vi "曲线.vi"() -> ()   [LabVIEW 2020]
uses:
  Global_Variable/Global.vi
  Database/Global1.vi
  Global_Variable/A131258.vi
  <vilib>/addons/database/Connection.llb/DB Tools Open Connec (String).vi
  <vilib>/addons/database/Connection.llb/Conn Execute.vi
  <vilib>/addons/database/Recordset.llb/Rec Fetch Recordset Data (R).vi
  <vilib>/Utility/config.llb/NI_LVConfig.lvlib
  <vilib>/addons/database/NI_Database_API.lvlib
panel:
  out "CODE_ID":string
  out "联机模式":string
  out "用户权限":string
  out "用户名":string
  in  "报表":string[][](table)=[["mm"], ["mm/s"]]
  in  "判定结果 3":bool[][](array[boolean])=[[TRUE]]
  in  "选项卡控件 2":enum32{"左工位压装曲线", "右工位压装曲线 ", "参数查看"}(tab)
  out "左压装下限":dbl format="%#.2f"
  out "左压装上限":dbl format="%#.2f"
  out "左下限2":dbl format="%#.2f"
  out "左上限2":dbl format="%#.2f"
  out "左下限1":dbl format="%#.2f"
  out "左上限1":dbl format="%#.2f"
  out "压装最大位移(mm)":dbl
  out "判定结果":bool
  out "力位移曲线":cluster{dbl[], dbl[]}[](graph)
  out "位移区间最大压力(KN)":dbl
  out "位移区间最小压力(KN)":dbl
  out "右位移下限":dbl format="%#.2f"
  out "右位移上限":dbl format="%#.2f"
  out "右下限2":dbl format="%#.2f"
  out "右上限2":dbl format="%#.2f"
  out "右下限1":dbl format="%#.2f"
  out "右上限1":dbl format="%#.2f"
  out "压装最大位移(mm) 2":dbl
  out "判定结果 2":bool
  out "力位移曲线 2":cluster{dbl[], dbl[]}[](graph)
  out "位移区间最大压力(KN) 2":dbl
  out "位移区间最小压力(KN) 2":dbl
  in  "删除":bool
  in  "确定":bool
  in  "添加":bool
  in  "退出":bool
  in  "更新":bool
  in  "产品型号":string(combo)
  in  "选项卡控件 3":enum32{"左工位参数", "右工位参数", "产品管理", "用户管理"}(tab)
  in  "左工位坐标轴参数":string[][](table)=[["mm"], ["mm/s"]]
  in  "左工位判定框参数":string[][](table)=[["mm"], ["mm/s"]]
  in  "左工位结果判定参数":string[][](table)=[["mm"], ["mm/s"]]
  in  "右工位结果判定参数":string[][](table)=[["mm"], ["mm/s"]]
  in  "右工位判定框参数":string[][](table)=[["mm"], ["mm/s"]]
  in  "右工位坐标轴参数":string[][](table)=[["mm"], ["mm/s"]]
  in  "请输入添加的产品名称":string
  in  "请选择要删除的产品":string(combo)
  in  "确定按钮":bool
  # "180上下柱管总成装配"
  # "上限"
  # "下限"
  # "上限"
  # "下限"
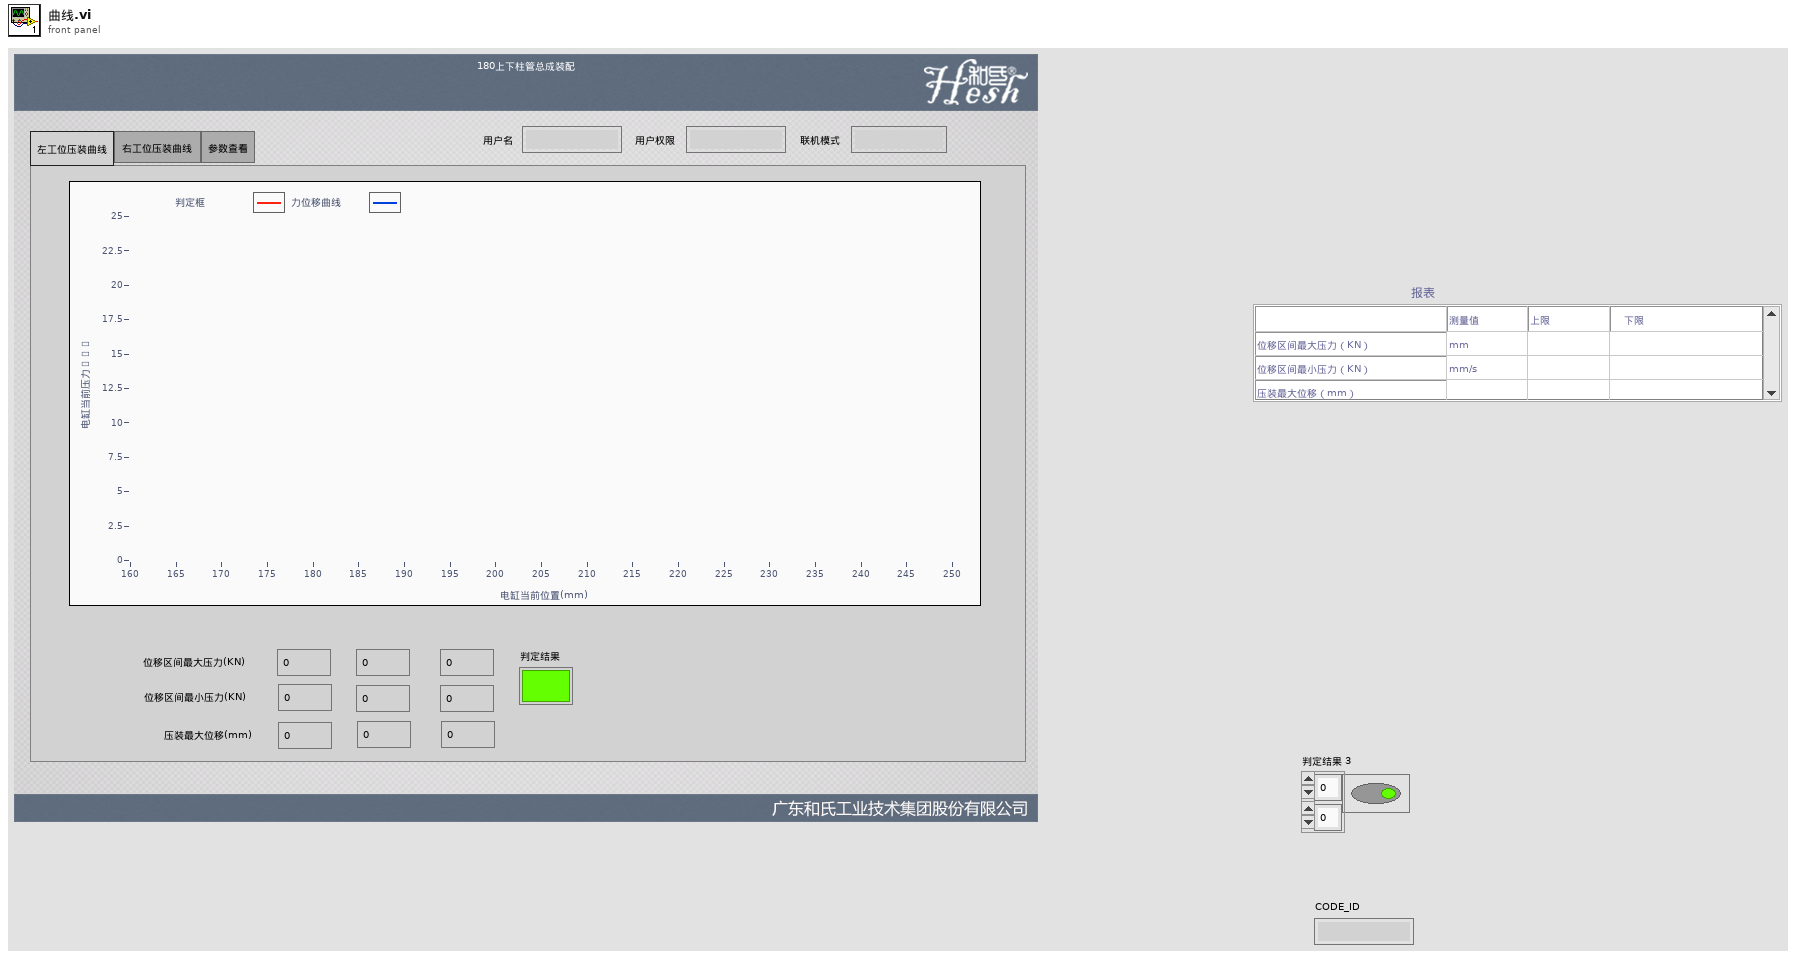
[diagram p1: front panel]
types:
  T1 = enum32{"Invalid", "Standard", "Closed", "Hidden", "Minimized", "Maximized"}
  T2 = cluster{"用户编号":string, "用户名":string, "用户密码(密文)":string, "用户权限":string}
  T3 = cluster{"设备名称":string, "用户名":string, "设备状态":enum16{"设备离线", "设备正常", "设备缺料", "设备故障", "质量报警"}, "附加信息":string}
  T4 = typedef "NI_LVConfig.lvlib/Config Data RefNum.ctl" = refnum<k1>
  T5 = typedef "NI_Database_API.lvlib/Conn ObjectReference.ctl" = refnum<k1>
  T6 = typedef "NI_Database_API.lvlib/Rec ObjectReference.ctl" = refnum<k1>
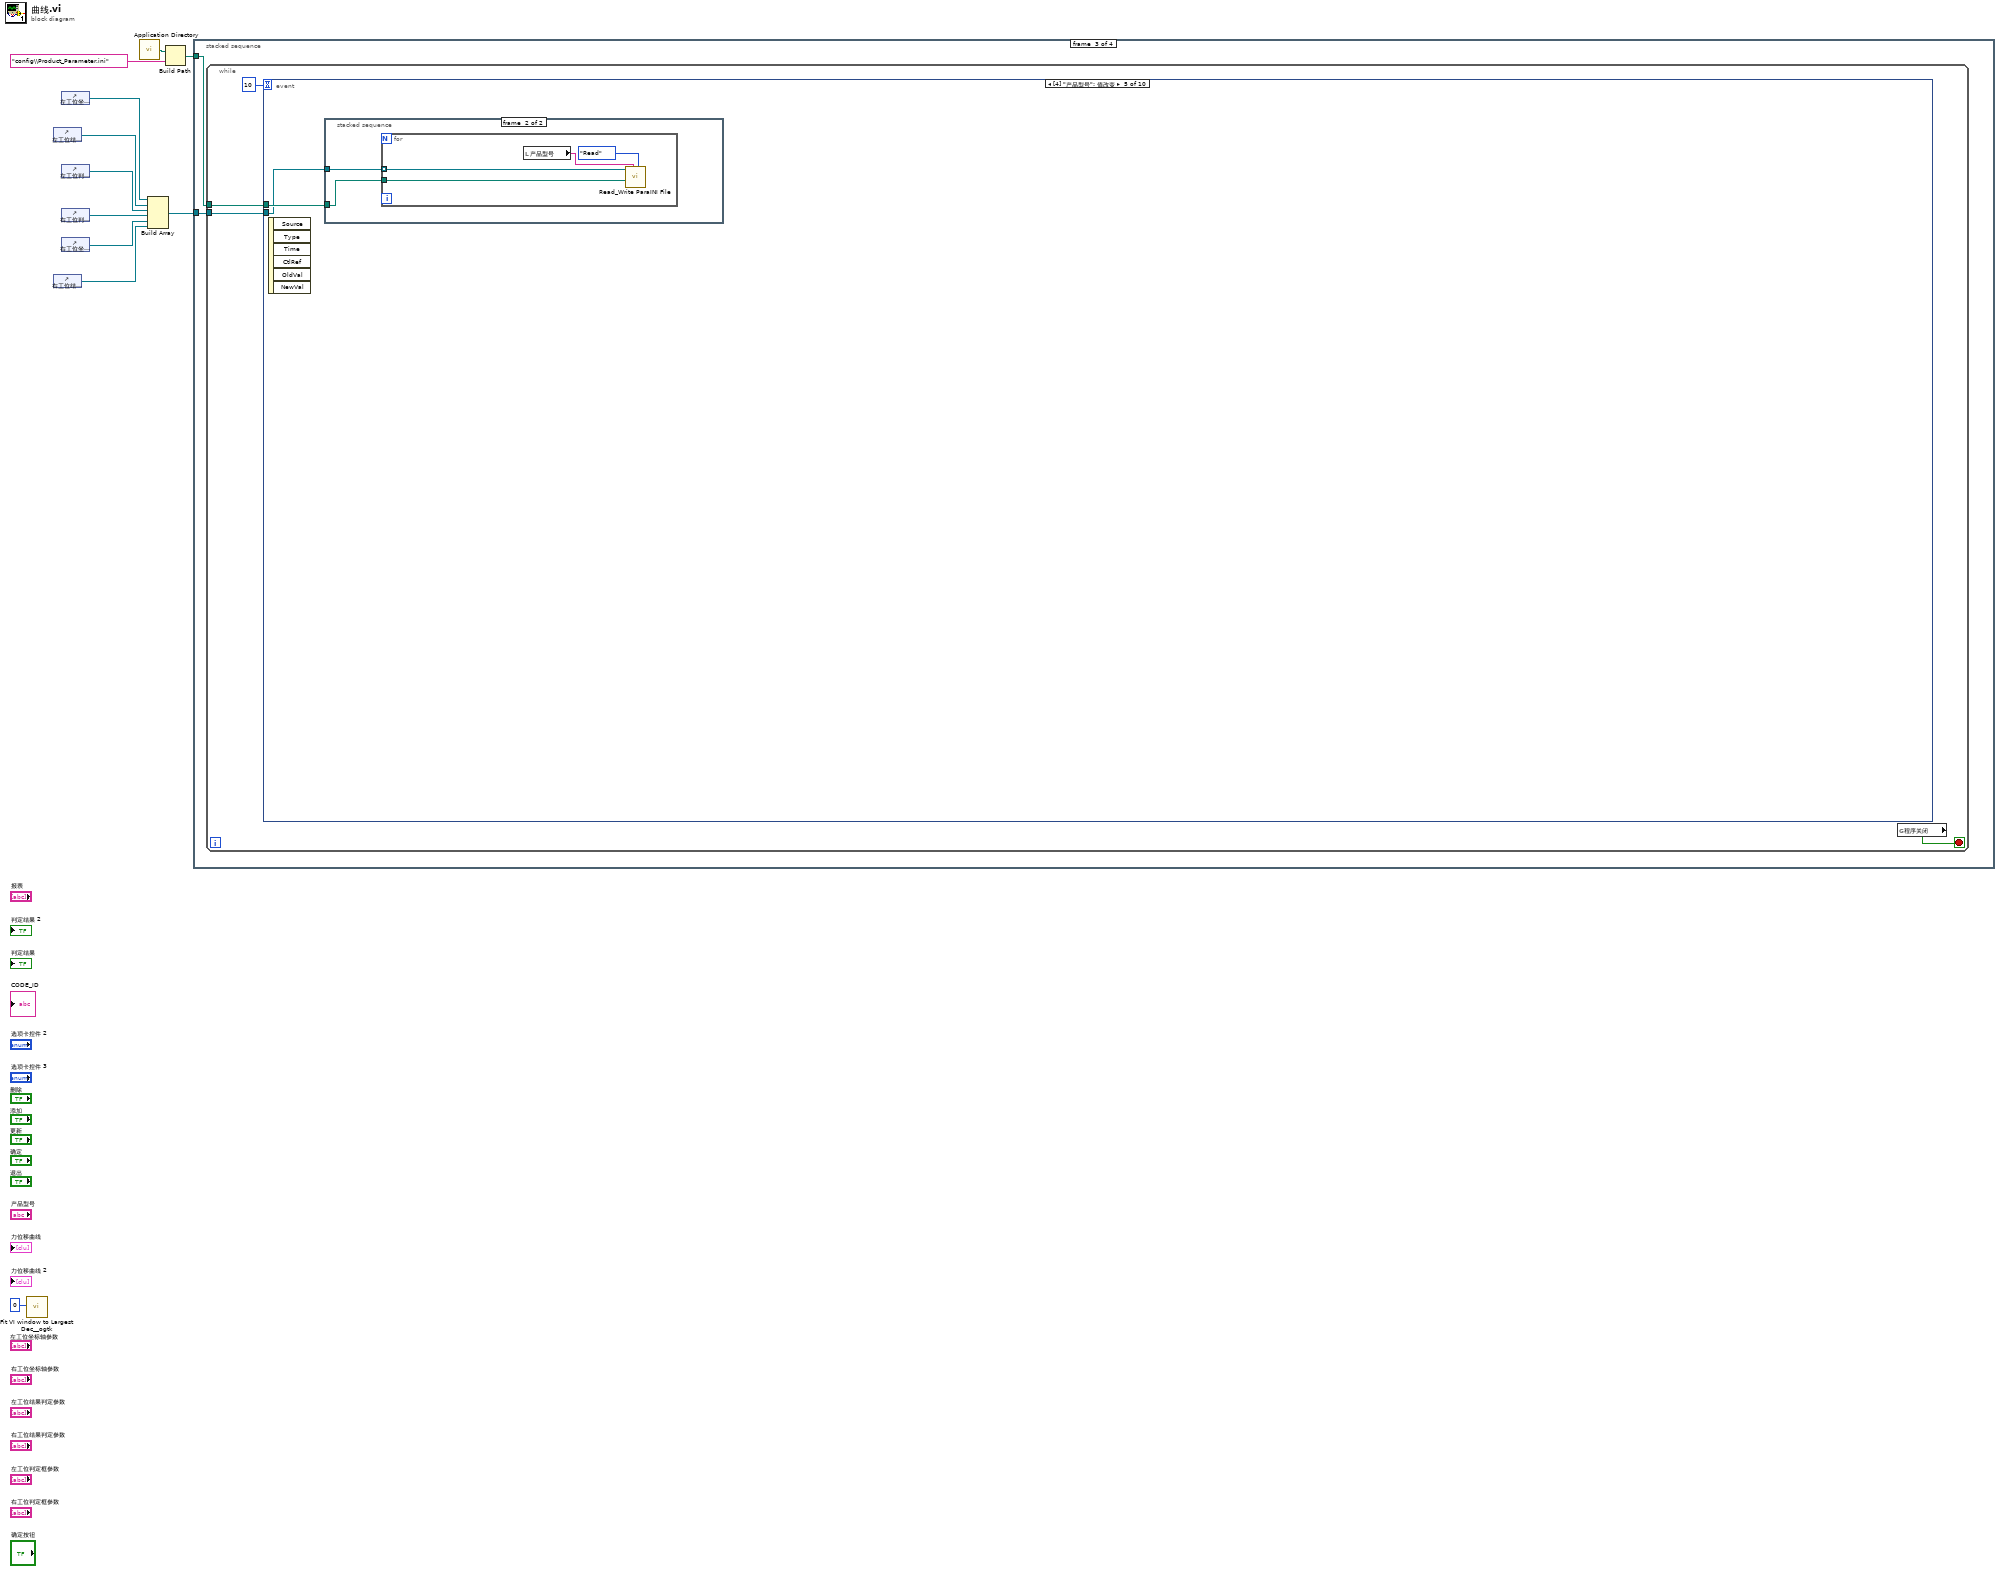
[diagram p0: block diagram]
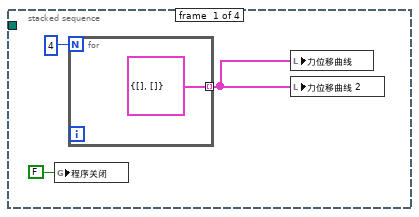
[diagram p2: hidden frame]
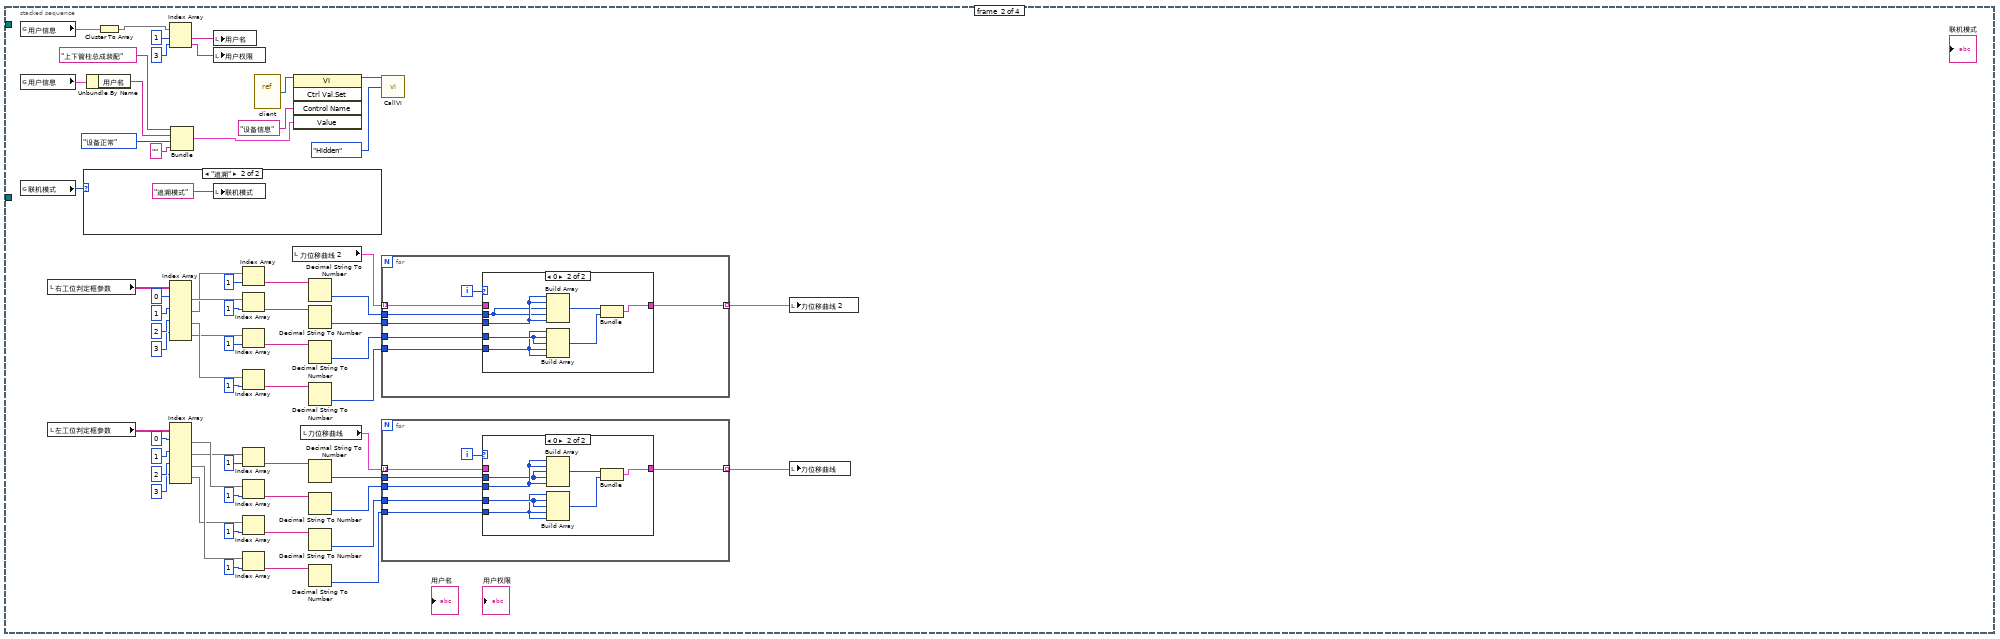
[diagram p3: hidden frame]
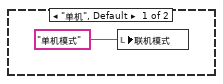
[diagram p4: hidden frame]
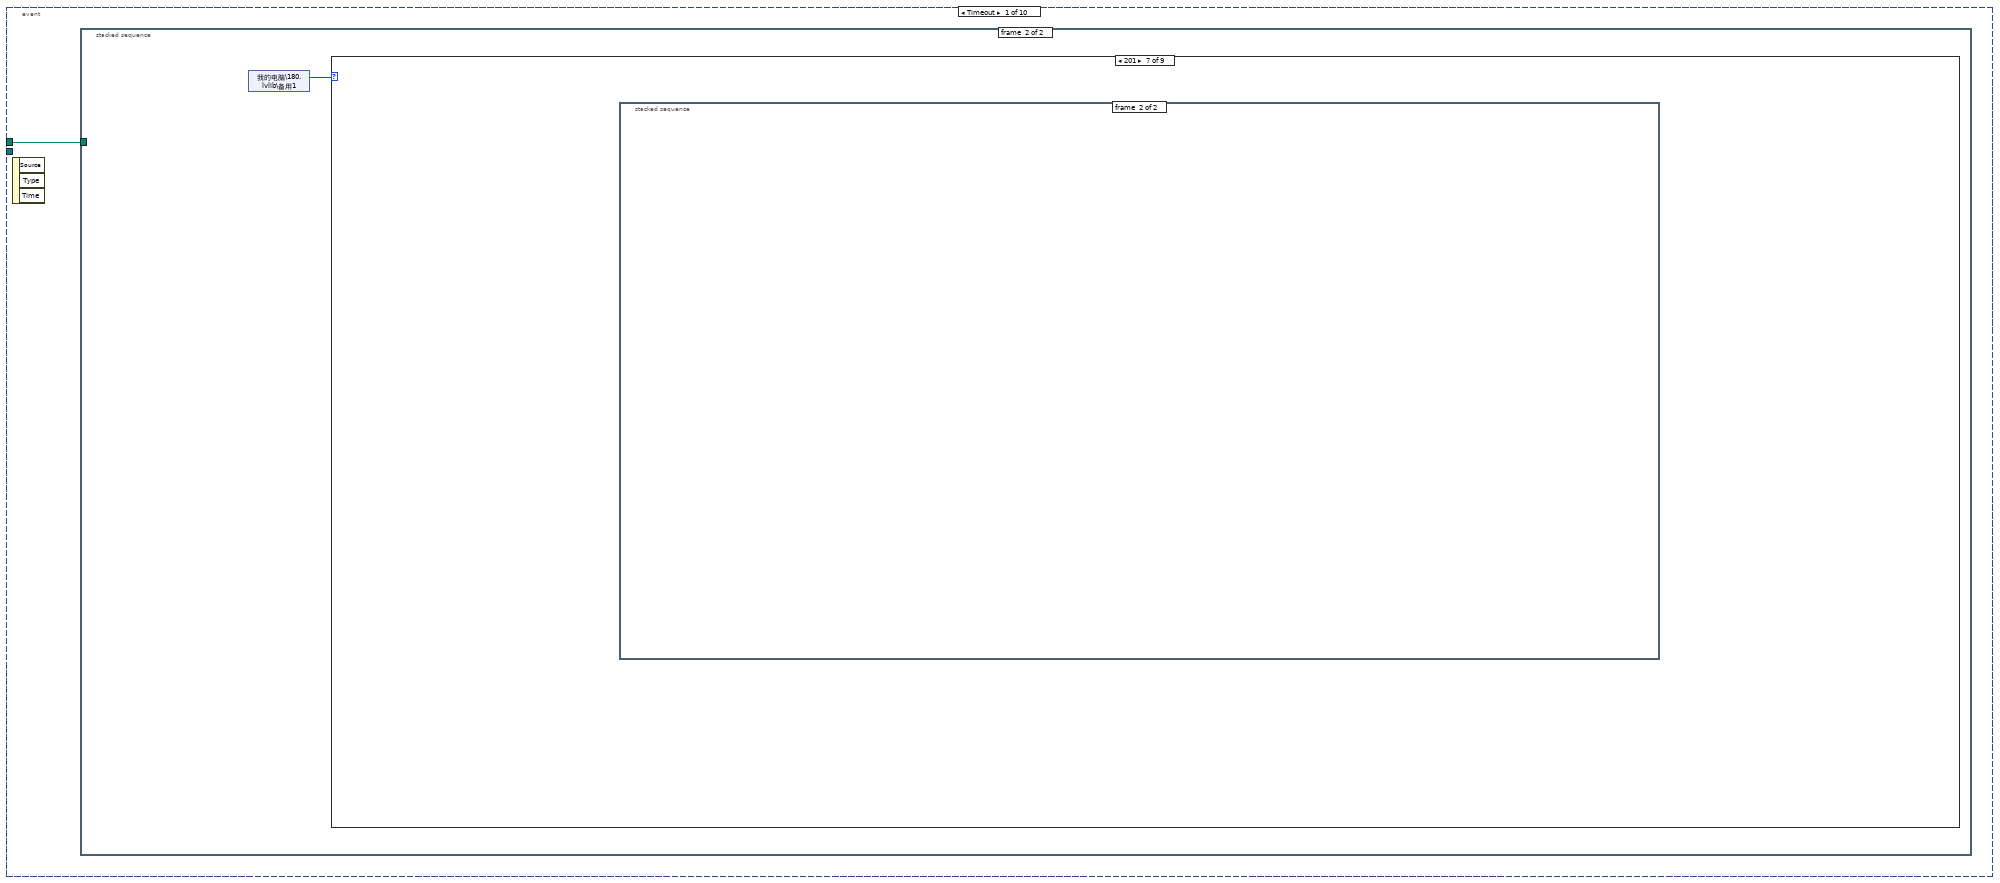
[diagram p7: hidden frame]
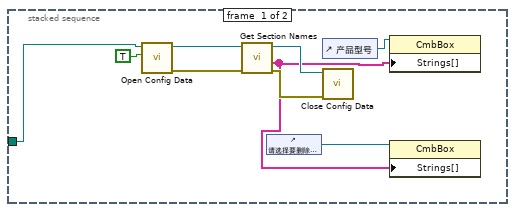
[diagram p8: hidden frame]
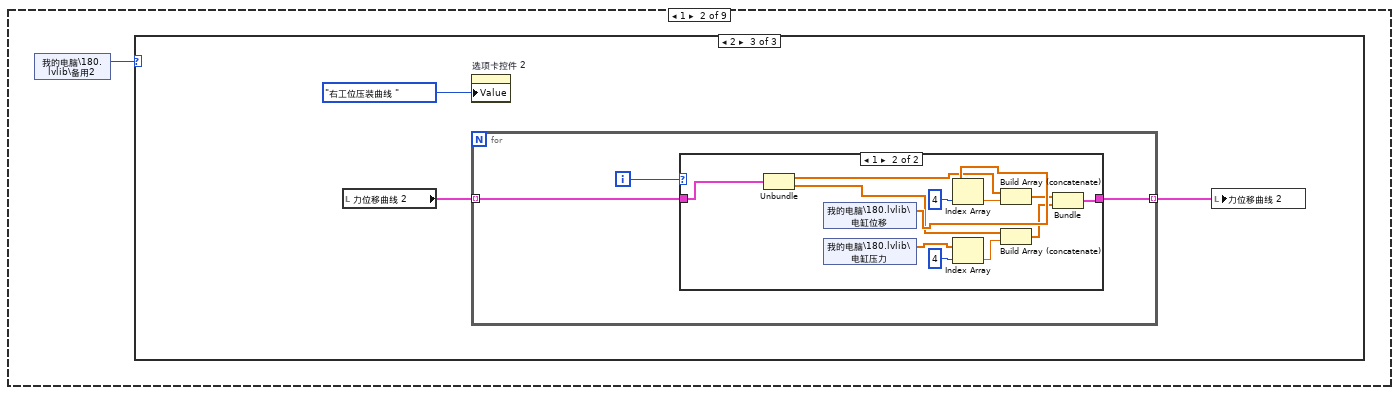
[diagram p10: hidden frame]
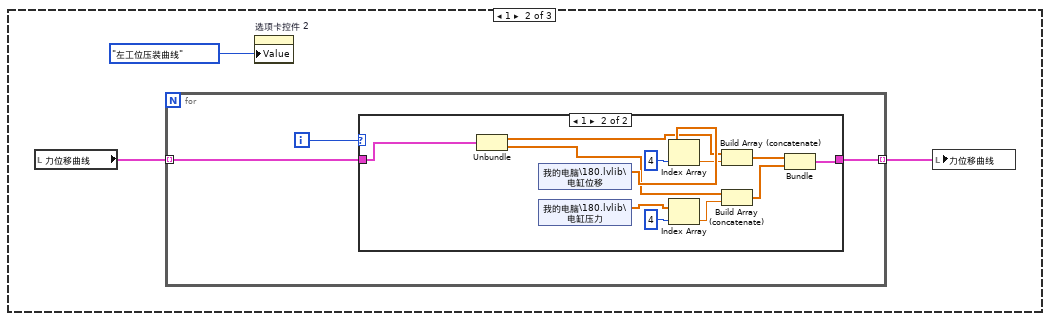
[diagram p12: hidden frame]
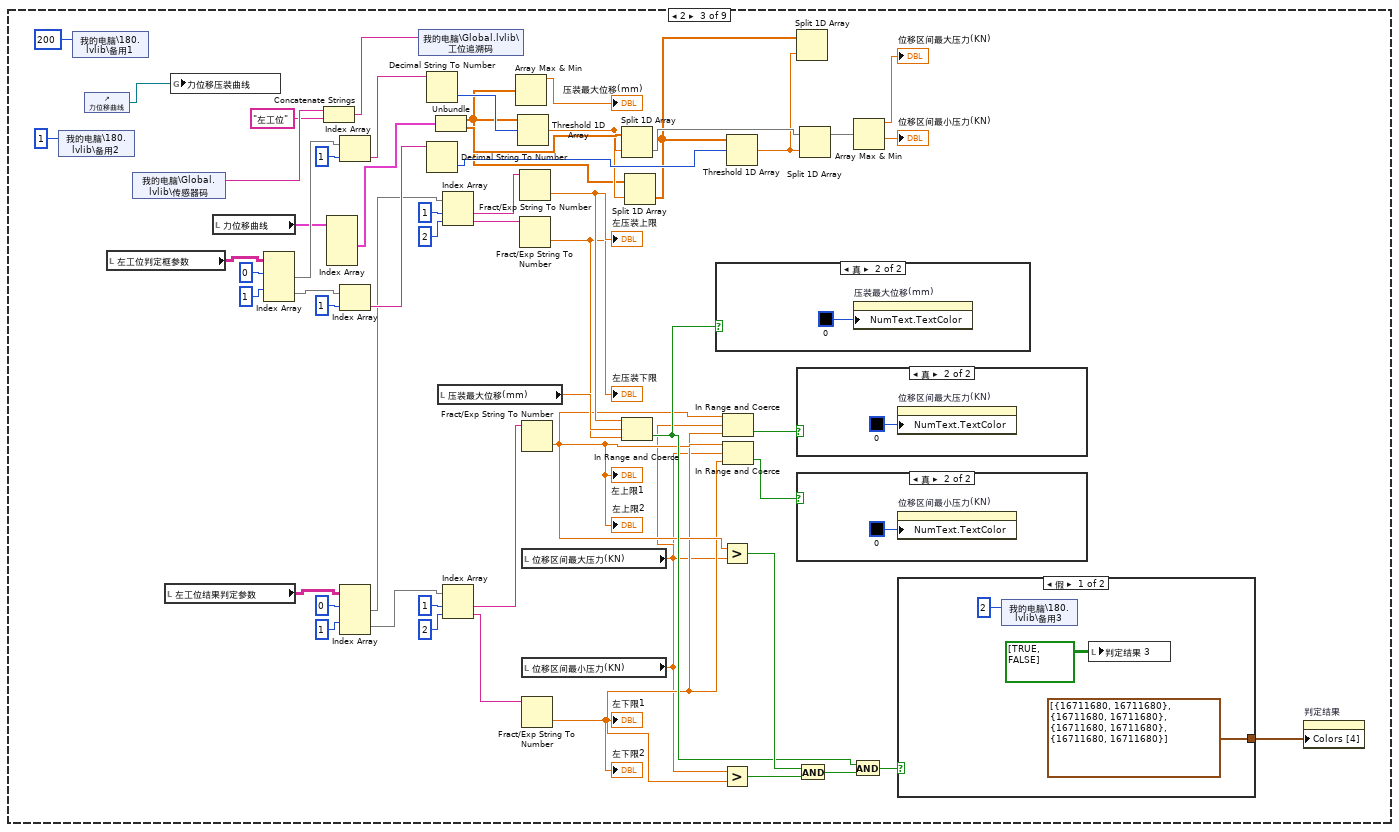
[diagram p15: hidden frame]
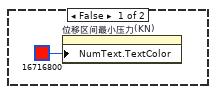
[diagram p16: hidden frame]
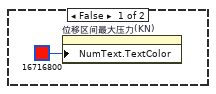
[diagram p17: hidden frame]
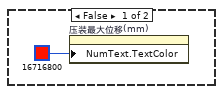
[diagram p18: hidden frame]
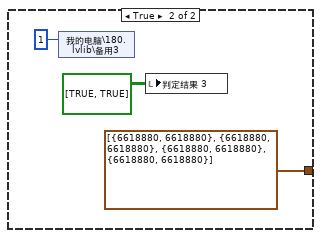
[diagram p19: hidden frame]
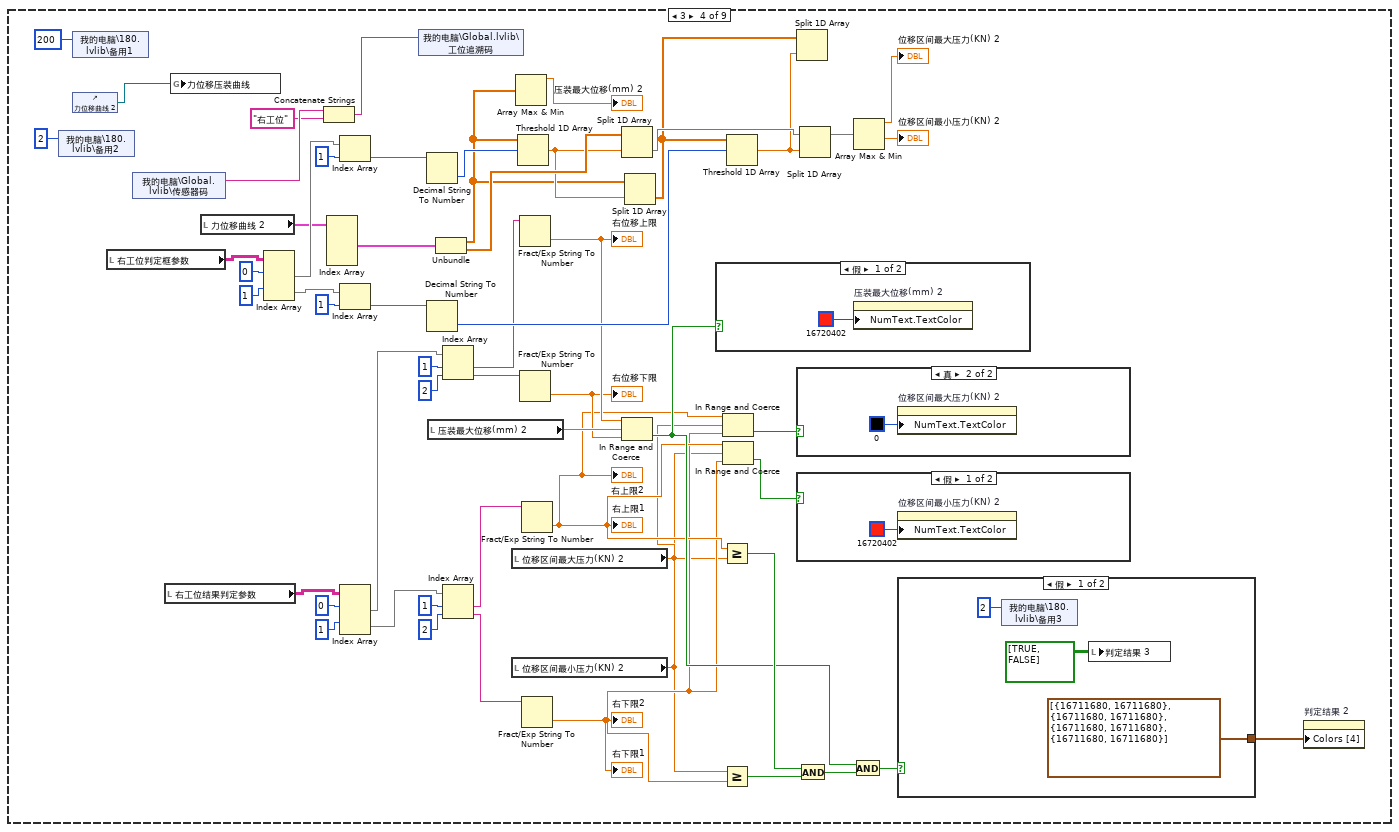
[diagram p20: hidden frame]
diagram:
  n1 = call "Fit VI window to Largest Dec__ogtk.vi"("border spacing (2 px)"=0) -> ()  [unwired: 5 in, 2 out]
  n2 = control-ref of="左工位结果判定参数"() -> (w5:refnum<vi>)
  n3 = control-ref of="右工位结果判定参数"() -> (w1:refnum<vi>)
  n4 = control-ref of="左工位坐标轴参数"() -> (w6:refnum<vi>)
  n5 = control-ref of="左工位判定框参数"() -> (w4:refnum<vi>)
  n6 = control-ref of="右工位判定框参数"() -> (w3:refnum<vi>)
  n7 = control-ref of="右工位坐标轴参数"() -> (w2:refnum<vi>)
  n8 = call <vilib>:"Application Directory.vi"() -> ("Application Directory"=w11:path)
  n9 = Build Array(w6, w5, w4, w3, w2, w1) -> (w7:refnum<vi>[])
  n10 = Build Path(base path=w11, name or relative path="config\\Product_Parameter.ini" ("名称或相对路径")) -> (appended path=w8:path)
  n11 = stacked-sequence {
    tunnel: w8 -> [_ _ w112 _]
    tunnel: w7 -> [_ _ w111 _]
    frame #0 {
      n12 = global write "Global.vi" "程序关闭"(FALSE ("程序关闭")) -> ()
      n13 = for {
        N: 4 -> [_]
        tunnel: [cluster{dbl[], dbl[]} {[], []}] -> w13 mode=indexing
      }
      n14 = local write "力位移曲线"(w13) -> ()
      n15 = local write "力位移曲线 2"(w13) -> ()
    }
    frame #1 {
      n16 = global read "Global1.vi" "用户信息"() -> (w32:T2)
      n17 = global read "Global1.vi" "用户信息"() -> (w23:T2)
      n18 = global read "Global1.vi" "联机模式"() -> (w26:enum16{"单机", "追溯"})
      n19 = local read "右工位判定框参数"() -> (w36:string[][])
      n20 = local read "左工位判定框参数"() -> (w33:string[][])
      n21 = case shown="\"追溯\"" w26 {
        frame "单机", Default {
          n22 = local write "联机模式"("单机模式" ("联机模式")) -> ()
        }
        frame "追溯" {
          n23 = local write "联机模式"("追溯模式" ("联机模式")) -> ()
        }
      }
      n24 = Unbundle By Name(w23) -> ("用户名"=w22:string)
      n25 = Cluster To Array(cluster=w32) -> (array=w31:string[])
      n26 = Index Array(array=w31, index #1=1 ("索引"), index #2=3 ("索引")) -> (element #1=w28:string, element #2=w27:string)
      n27 = Index Array(array=w36, index (row) #1=0 ("索引 (行)"), index (row) #2=1 ("索引 (行)"), index (row) #3=2 ("索引 (行)"), index (row) #4=3 ("索引 (行)")) -> (element #1=w52:string[], element #2=w47:string[], element #3=w46:string[], element #4=w45:string[])  [unwired: 4 in]
      n28 = Index Array(array=w33, index (row) #1=0 ("索引 (行)"), index (row) #2=1 ("索引 (行)"), index (row) #3=2 ("索引 (行)"), index (row) #4=3 ("索引 (行)")) -> (element #1=w74:string[], element #2=w69:string[], element #3=w68:string[], element #4=w67:string[])  [unwired: 4 in]
      n29 = Bundle("设备名称"="上下管柱总成装配", "用户名"=w22, "设备状态"=enum16{"设备离线", "设备正常", "设备缺料", "设备故障", "质量报警"}."设备正常", "附加信息"="") -> (w21:T3)  [unwired: 1 in]
      n30 = local write "用户名"(w28) -> ()
      n31 = local write "用户权限"(w27) -> ()
      n32 = Index Array(array=w47, index=1 ("索引")) -> (element=w39:string)
      n33 = Index Array(array=w52, index=1 ("索引")) -> (element=w40:string)
      n34 = Index Array(array=w45, index=1 ("索引")) -> (element=w37:string)
      n35 = Index Array(array=w46, index=1 ("索引")) -> (element=w38:string)
      n36 = Index Array(array=w69, index=1 ("索引")) -> (element=w61:string)
      n37 = Index Array(array=w74, index=1 ("索引")) -> (element=w62:string)
      n38 = Index Array(array=w67, index=1 ("索引")) -> (element=w59:string)
      n39 = Index Array(array=w68, index=1 ("索引")) -> (element=w60:string)
      n40 = vi-ref "client.vi"() -> (w25:refnum<vi>)
      n41 = local read "力位移曲线 2"() -> (w35:cluster{dbl[], dbl[]}[])
      n42 = invoke class="VI" method="Ctrl Val.Set"(reference=w25, "Control Name"="设备信息" ("控件名"), "Value"=w21) -> (reference out=w24:refnum<vi>)  [unwired: 2 in, 4 out]
      n43 = local read "力位移曲线"() -> (w57:cluster{dbl[], dbl[]}[])
      n44 = Decimal String To Number(string=w39) -> (number=w43:i32)  [unwired: 2 in, 1 out]
      n45 = Decimal String To Number(string=w40) -> (number=w44:i32)  [unwired: 2 in, 1 out]
      n46 = Decimal String To Number(string=w37) -> (number=w42:i32)  [unwired: 2 in, 1 out]
      n47 = Decimal String To Number(string=w38) -> (number=w41:i32)  [unwired: 2 in, 1 out]
      n48 = Decimal String To Number(string=w61) -> (number=w65:i32)  [unwired: 2 in, 1 out]
      n49 = Decimal String To Number(string=w62) -> (number=w66:i32)  [unwired: 2 in, 1 out]
      n50 = Decimal String To Number(string=w59) -> (number=w64:i32)  [unwired: 2 in, 1 out]
      n51 = Decimal String To Number(string=w60) -> (number=w63:i32)  [unwired: 2 in, 1 out]
      n52 = call "CallVI.vi"("VI引用"=w24, "状态"=T1."Hidden") -> ()  [unwired: 11 in, 3 out]
      n53 = for {
        tunnel: [w87] -> w34 mode=indexing
        tunnel: w35 -> [w86] mode=indexing
        tunnel: w44 -> [w84]
        tunnel: w43 -> [w83]
        tunnel: w42 -> [w82]
        tunnel: w41 -> [w81]
        i -> [w85]
        n54 = case shown="0" w85 {
          tunnel: [w88 w93] -> w87
          tunnel: w86 -> [w88 _]
          tunnel: w84 -> [_ w92]
          tunnel: w83 -> [_ w91]
          tunnel: w82 -> [_ w90]
          tunnel: w81 -> [_ w89]
          frame Default {
          }
          frame 0 {
            n55 = Build Array(w92, w92, w91, w91, w92) -> (w94:i32[])
            n56 = Build Array(w89, w90, w90, w89, w89) -> (w95:i32[])
            n57 = Bundle(w94, w95) -> (w93:cluster{i32[], i32[]})  [unwired: 1 in]
          }
        }
      }
      n58 = for {
        tunnel: [w102] -> w58 mode=indexing
        tunnel: w57 -> [w101] mode=indexing
        tunnel: w66 -> [w99]
        tunnel: w65 -> [w98]
        tunnel: w64 -> [w97]
        tunnel: w63 -> [w96]
        i -> [w100]
        n59 = case shown="0" w100 {
          tunnel: [w103 w108] -> w102
          tunnel: w101 -> [w103 _]
          tunnel: w99 -> [_ w107]
          tunnel: w98 -> [_ w106]
          tunnel: w97 -> [_ w105]
          tunnel: w96 -> [_ w104]
          frame Default {
          }
          frame 0 {
            n60 = Build Array(w107, w107, w106, w106, w107) -> (w109:i32[])
            n61 = Build Array(w104, w105, w105, w104, w104) -> (w110:i32[])
            n62 = Bundle(w109, w110) -> (w108:cluster{i32[], i32[]})  [unwired: 1 in]
          }
        }
      }
      n63 = local write "力位移曲线 2"(w34) -> ()
      n64 = local write "力位移曲线"(w58) -> ()
    }
    frame #2 {
      n65 = while {
        tunnel: w112 -> [w115]
        tunnel: w111 -> [w114]
        stop <- w113 stop-if-true
        n66 = event shown="[4] \"产品型号\": 值改变" {
          selector: _ -> [_ _ _ _ _ _ _ _ _ _]
          dyn-events: _ -> [_ _ _ _ _ _ _ _ _ _]
          timeout: 10 -> [_ _ _ _ _ _ _ _ _ _]
          tunnel: w115 -> [w117 w496 _ w637 w656 _ w667 _ _ _]
          tunnel: w114 -> [_ _ _ w636 w655 _ w666 _ _ _]
          event Timeout {
            n67 = event-data() -> ()  [unwired: 1 in, 3 out]
            n68 = stacked-sequence {
              tunnel: w117 -> [w118 _]
              frame #0 {
                n69 = call <vilib>:"Open Config Data.vi"("create file if necessary (T)"=TRUE, "configuration file path"=w118) -> ("error out"=w123:errorcluster, "refnum"=w122:T4)  [unwired: 7 in, 1 out]
                n70 = call <vilib>:"Get Section Names.vi"("error in (no error)"=w123, "refnum"=w122) -> ("error out"=w125:errorcluster, "section names"=w121:string[], "refnum out"=w124:T4)  [unwired: 7 in]
                n71 = control-ref of="请选择要删除的产品"() -> (w119:refnum<vi>)
                n72 = control-ref of="产品型号"() -> (w120:refnum<vi>)
                n73 = call <vilib>:"Close Config Data.vi"("error in (no error)"=w125, "refnum"=w124) -> ()  [unwired: 8 in, 2 out]
                n74 = property on="属性节点" class="CmbBox"(reference=w120, "Strings[]"=w121) -> ()  [unwired: 1 in, 2 out]
                n75 = property on="属性节点" class="CmbBox"(reference=w119, "Strings[]"=w121) -> ()  [unwired: 1 in, 2 out]
              }
              frame #1 {
                n76 = shared-variable "我的电脑\\180.lvlib\\备用1"() -> (w127:u16)  [unwired: 1 in, 1 out]
                n77 = case shown="201" w127 {
                  frame 0, Default {
                  }
                  frame 1 {
                    n78 = shared-variable "我的电脑\\180.lvlib\\备用2"() -> (w128:u16)  [unwired: 1 in, 1 out]
                    n79 = case shown="2" w128 {
                      frame 0, Default {
                      }
                      frame 1 {
                        n80 = local read "力位移曲线"() -> (w130:cluster{dbl[], dbl[]}[])
                        n81 = for {
                          tunnel: [w134] -> w129 mode=indexing
                          tunnel: w130 -> [w133] mode=indexing
                          i -> [w132]
                          n82 = case shown="1" w132 {
                            tunnel: [w135 w139] -> w134
                            tunnel: w133 -> [w135 w138]
                            frame Default {
                            }
                            frame 1 {
                              n83 = Unbundle(w138) -> (w143:dbl[], w142:dbl[])
                              n84 = shared-variable "我的电脑\\180.lvlib\\电缸位移"() -> (w145:sgl[])  [unwired: 1 in, 1 out]
                              n85 = shared-variable "我的电脑\\180.lvlib\\电缸压力"() -> (w147:sgl[])  [unwired: 1 in, 1 out]
                              n86 = Index Array(array=w145, index=4) -> (element=w136:sgl)
                              n87 = Index Array(array=w147, index=4) -> (element=w137:sgl)
                              n88 = Build Array (concatenate)(w143, w136) -> (w141:dbl[])
                              n89 = Build Array (concatenate)(w142, w137) -> (w140:dbl[])
                              n90 = Bundle(w141, w140) -> (w139:cluster{dbl[], dbl[]})  [unwired: 1 in]
                            }
                          }
                        }
                        n91 = property on="选项卡控件 2" class="TabCtl (严格)"("Value"=enum32{"左工位压装曲线", "右工位压装曲线 ", "参数查看"}."左工位压装曲线" ("选项卡控件 2")) -> ()  [unwired: 2 in, 2 out]
                        n92 = local write "力位移曲线"(w129) -> ()
                      }
                      frame 2 {
                        n93 = local read "力位移曲线 2"() -> (w149:cluster{dbl[], dbl[]}[])
                        n94 = property on="选项卡控件 2" class="TabCtl (严格)"("Value"=enum32{"左工位压装曲线", "右工位压装曲线 ", "参数查看"}."右工位压装曲线 " ("选项卡控件 2")) -> ()  [unwired: 2 in, 2 out]
                        n95 = for {
                          tunnel: [w153] -> w150 mode=indexing
                          tunnel: w149 -> [w152] mode=indexing
                          i -> [w151]
                          n96 = case shown="1" w151 {
                            tunnel: [w154 w158] -> w153
                            tunnel: w152 -> [w154 w157]
                            frame Default {
                            }
                            frame 1 {
                              n97 = Unbundle(w157) -> (w162:dbl[], w161:dbl[])
                              n98 = shared-variable "我的电脑\\180.lvlib\\电缸位移"() -> (w164:sgl[])  [unwired: 1 in, 1 out]
                              n99 = shared-variable "我的电脑\\180.lvlib\\电缸压力"() -> (w166:sgl[])  [unwired: 1 in, 1 out]
                              n100 = Index Array(array=w164, index=4) -> (element=w155:sgl)
                              n101 = Index Array(array=w166, index=4) -> (element=w156:sgl)
                              n102 = Build Array (concatenate)(w162, w155) -> (w160:dbl[])
                              n103 = Build Array (concatenate)(w161, w156) -> (w159:dbl[])
                              n104 = Bundle(w160, w159) -> (w158:cluster{dbl[], dbl[]})  [unwired: 1 in]
                            }
                          }
                        }
                        n105 = local write "力位移曲线 2"(w150) -> ()
                      }
                    }
                  }
                  frame 2 {
                    n106 = shared-variable "我的电脑\\180.lvlib\\备用2"(u16 1 ("备用1")) -> ()  [unwired: 1 in, 1 out]
                    n107 = shared-variable "我的电脑\\180.lvlib\\备用1"(u16 200 ("备用1")) -> ()  [unwired: 1 in, 1 out]
                    n108 = control-ref of="力位移曲线"() -> (w172:refnum<vi>)
                    n109 = local read "左工位判定框参数"() -> (w222:string[][])
                    n110 = shared-variable "我的电脑\\Global.lvlib\\传感器码"() -> (w170:string)  [unwired: 1 in, 1 out]
                    n111 = local read "左工位结果判定参数"() -> (w194:string[][])
                    n112 = global write "A131258.vi" "力位移压装曲线"(w172) -> ()
                    n113 = local read "力位移曲线"() -> (w217:cluster{dbl[], dbl[]}[])
                    n114 = Index Array(array=w222, index (row) #1=0 ("索引 (行)"), index (row) #2=1 ("索引 (行)")) -> (element #1=w218:string[], element #2=w219:string[])  [unwired: 2 in]
                    n115 = Concatenate Strings(w170, "左工位" ("字符串")) -> (w171:string)
                    n116 = Index Array(array=w217) -> (element #2=w216:cluster{dbl[], dbl[]})  [unwired: 4 in, 3 out]
                    n117 = Index Array(array=w218, index=1 ("索引")) -> (element=w220:string)
                    n118 = Index Array(array=w219, index=1 ("索引")) -> (element=w221:string)
                    n119 = Index Array(array=w194, index (row) #1=0 ("索引 (行)"), index (row) #2=1 ("索引 (行)")) -> (element #1=w195:string[], element #2=w200:string[])  [unwired: 2 in]
                    n120 = shared-variable "我的电脑\\Global.lvlib\\工位追溯码"(w171) -> ()  [unwired: 1 in, 1 out]
                    n121 = Decimal String To Number(string=w220) -> (number=w203:i32)  [unwired: 2 in, 1 out]
                    n122 = Decimal String To Number(string=w221) -> (number=w223:i32)  [unwired: 2 in, 1 out]
                    n123 = Unbundle(w216) -> (w201:dbl[], w215:dbl[])
                    n124 = local read "压装最大位移(mm)"() -> (w191:dbl)
                    n125 = Index Array(array=w195, index #1=1 ("索引"), index #2=2 ("索引")) -> (element #1=w190:string, element #2=w189:string)
                    n126 = Index Array(array=w200, index #1=1 ("索引"), index #2=2 ("索引")) -> (element #1=w188:string, element #2=w187:string)
                    n127 = Array Max & Min(array=w201) -> (max value=→"压装最大位移(mm)":dbl)  [unwired: 3 out]
                    n128 = Threshold 1D Array(2:w203, 3:w201) -> (0:w214:dbl)  [unwired: 1 in]
                    n129 = Fract/Exp String To Number(string=w190) -> (number=w181:dbl)  [unwired: 3 in, 1 out]
                    "左压装上限" <- w181
                    n130 = Fract/Exp String To Number(string=w189) -> (number=w180:dbl)  [unwired: 3 in, 1 out]
                    "左压装下限" <- w180
                    n131 = Fract/Exp String To Number(string=w188) -> (number=w176:dbl)  [unwired: 3 in, 1 out]
                    "左上限1" <- w176
                    "左上限2" <- w176
                    n132 = local read "位移区间最大压力(KN)"() -> (w174:dbl)
                    n133 = local read "位移区间最小压力(KN)"() -> (w173:dbl)
                    n134 = Fract/Exp String To Number(string=w187) -> (number=w175:dbl)  [unwired: 3 in, 1 out]
                    "左下限1" <- w175
                    "左下限2" <- w175
                    n135 = Split 1D Array(array=w215, index=w214) -> (second subarray=w213:dbl[])  [unwired: 1 out]
                    n136 = In Range and Coerce(upper limit=w181, x=w191, lower limit=w180) -> (In Range?=w179:bool)  [unwired: 1 out]
                    n137 = Split 1D Array(array=w201, index=w214) -> (second subarray=w212:dbl[])  [unwired: 1 out]
                    n138 = case shown="真" w179 {
                      frame False {
                        n139 = property on="压装最大位移(mm)" class="DigNum (严格)"("NumText.TextColor"=u32 16716800) -> ()  [unwired: 2 in, 2 out]
                      }
                      frame True {
                        n140 = property on="压装最大位移(mm)" class="DigNum (严格)"("NumText.TextColor"=u32 0) -> ()  [unwired: 2 in, 2 out]
                      }
                    }
                    n141 = Greater?(x=w176, y=w174) -> (0:w186:bool)
                    n142 = Greater?(x=w173, y=w175) -> (0:w185:bool)
                    n143 = In Range and Coerce(upper limit=w176, x=w174, lower limit=w175) -> (In Range?=w178:bool)  [unwired: 1 out]
                    n144 = In Range and Coerce(upper limit=w176, x=w173, lower limit=w175) -> (In Range?=w177:bool)  [unwired: 1 out]
                    n145 = Threshold 1D Array(2:w223, 3:w212) -> (0:w211:dbl)  [unwired: 1 in]
                    n146 = Split 1D Array(array=w212, index=w211) -> ()  [unwired: 2 out]
                    n147 = case shown="真" w178 {
                      frame False {
                        n148 = property on="位移区间最大压力(KN)" class="DigNum (严格)"("NumText.TextColor"=u32 16716800) -> ()  [unwired: 2 in, 2 out]
                      }
                      frame True {
                        n149 = property on="位移区间最大压力(KN)" class="DigNum (严格)"("NumText.TextColor"=u32 0) -> ()  [unwired: 2 in, 2 out]
                      }
                    }
                    n150 = case shown="真" w177 {
                      frame False {
                        n151 = property on="位移区间最小压力(KN)" class="DigNum (严格)"("NumText.TextColor"=u32 16716800) -> ()  [unwired: 2 in, 2 out]
                      }
                      frame True {
                        n152 = property on="位移区间最小压力(KN)" class="DigNum (严格)"("NumText.TextColor"=u32 0) -> ()  [unwired: 2 in, 2 out]
                      }
                    }
                    n153 = And(x=w186, y=w185) -> (x .and. y?=w184:bool)
                    n154 = Split 1D Array(array=w213, index=w211) -> (first subarray=w210:dbl[])  [unwired: 1 out]
                    n155 = And(x=w179, y=w184) -> (x .and. y?=w183:bool)
                    n156 = Array Max & Min(array=w210) -> (max value=→"位移区间最大压力(KN)":dbl, min value=→"位移区间最小压力(KN)":dbl)  [unwired: 2 out]
                    n157 = case shown="假" w183 {
                      tunnel: [cluster{u32, u32}[] [{16711680, 16711680}, {16711680, 16711680}, {16711680, 16711680}, {16711680, 16711680}] cluster{u32, u32}[] [{6618880, 6618880}, {6618880, 6618880}, {6618880, 6618880}, {6618880, 6618880}]] -> w182
                      frame False {
                        n158 = shared-variable "我的电脑\\180.lvlib\\备用3"(u16 2 ("备用1")) -> ()  [unwired: 1 in, 1 out]
                        n159 = local write "判定结果 3"(bool[][] [[TRUE, FALSE]] ("判定结果")) -> ()
                      }
                      frame True {
                        n160 = shared-variable "我的电脑\\180.lvlib\\备用3"(u16 1 ("备用1")) -> ()  [unwired: 1 in, 1 out]
                        n161 = local write "判定结果 3"(bool[][] [[TRUE, TRUE]] ("判定结果")) -> ()
                      }
                    }
                    n162 = property on="判定结果" class="Bool (严格)"("Colors [4]"=w182) -> ()  [unwired: 2 in, 2 out]
                  }
                  frame 3 {
                    n163 = shared-variable "我的电脑\\180.lvlib\\备用2"(u16 2 ("备用1")) -> ()  [unwired: 1 in, 1 out]
                    n164 = shared-variable "我的电脑\\180.lvlib\\备用1"(u16 200 ("备用1")) -> ()  [unwired: 1 in, 1 out]
                    n165 = control-ref of="力位移曲线 2"() -> (w241:refnum<vi>)
                    n166 = local read "右工位判定框参数"() -> (w278:string[][])
                    n167 = shared-variable "我的电脑\\Global.lvlib\\传感器码"() -> (w239:string)  [unwired: 1 in, 1 out]
                    n168 = local read "右工位结果判定参数"() -> (w271:string[][])
                    n169 = global write "A131258.vi" "力位移压装曲线"(w241) -> ()
                    n170 = local read "力位移曲线 2"() -> (w279:cluster{dbl[], dbl[]}[])
                    n171 = Index Array(array=w278, index (row) #1=0 ("索引 (行)"), index (row) #2=1 ("索引 (行)")) -> (element #1=w288:string[], element #2=w289:string[])  [unwired: 2 in]
                    n172 = Concatenate Strings(w239, "右工位" ("字符串")) -> (w240:string)
                    n173 = Index Array(array=w279) -> (element #2=w287:cluster{dbl[], dbl[]})  [unwired: 4 in, 3 out]
                    n174 = Index Array(array=w288, index=1 ("索引")) -> (element=w290:string)
                    n175 = Index Array(array=w289, index=1 ("索引")) -> (element=w291:string)
                    n176 = Index Array(array=w271, index (row) #1=0 ("索引 (行)"), index (row) #2=1 ("索引 (行)")) -> (element #1=w272:string[], element #2=w273:string[])  [unwired: 2 in]
                    n177 = shared-variable "我的电脑\\Global.lvlib\\工位追溯码"(w240) -> ()  [unwired: 1 in, 1 out]
                    n178 = Decimal String To Number(string=w290) -> (number=w276:i32)  [unwired: 2 in, 1 out]
                    n179 = Decimal String To Number(string=w291) -> (number=w292:i32)  [unwired: 2 in, 1 out]
                    n180 = local read "压装最大位移(mm) 2"() -> (w266:dbl)
                    n181 = Unbundle(w287) -> (w274:dbl[], w286:dbl[])
                    n182 = Index Array(array=w272, index #1=1 ("索引"), index #2=2 ("索引")) -> (element #1=w270:string, element #2=w267:string)
                    n183 = Index Array(array=w273, index #1=1 ("索引"), index #2=2 ("索引")) -> (element #1=w269:string, element #2=w268:string)
                    n184 = local read "位移区间最大压力(KN) 2"() -> (w253:dbl)
                    n185 = local read "位移区间最小压力(KN) 2"() -> (w252:dbl)
                    n186 = Array Max & Min(array=w274) -> (max value=→"压装最大位移(mm) 2":dbl)  [unwired: 3 out]
                    n187 = Threshold 1D Array(2:w276, 3:w274) -> (0:w277:dbl)  [unwired: 1 in]
                    n188 = Fract/Exp String To Number(string=w270) -> (number=w261:dbl)  [unwired: 3 in, 1 out]
                    "右位移上限" <- w261
                    n189 = Fract/Exp String To Number(string=w267) -> (number=w260:dbl)  [unwired: 3 in, 1 out]
                    "右位移下限" <- w260
                    n190 = Fract/Exp String To Number(string=w269) -> (number=w255:dbl)  [unwired: 3 in, 1 out]
                    "右上限1" <- w255
                    "右上限2" <- w255
                    n191 = Fract/Exp String To Number(string=w268) -> (number=w254:dbl)  [unwired: 3 in, 1 out]
                    "右下限1" <- w254
                    "右下限2" <- w254
                    n192 = Split 1D Array(array=w286, index=w277) -> (second subarray=w285:dbl[])  [unwired: 1 out]
                    n193 = In Range and Coerce(upper limit=w261, x=w266, lower limit=w260) -> (In Range?=w258:bool)  [unwired: 1 out]
                    n194 = Split 1D Array(array=w274, index=w277) -> (second subarray=w284:dbl[])  [unwired: 1 out]
                    n195 = case shown="假" w258 {
                      frame False {
                        n196 = property on="压装最大位移(mm) 2" class="DigNum (严格)"("NumText.TextColor"=u32 16720402) -> ()  [unwired: 2 in, 2 out]
                      }
                      frame True {
                        n197 = property on="压装最大位移(mm) 2" class="DigNum (严格)"("NumText.TextColor"=u32 0) -> ()  [unwired: 2 in, 2 out]
                      }
                    }
                    n198 = Greater Or Equal?(x=w255, y=w253) -> (x >= y?=w259:bool)
                    n199 = Greater Or Equal?(x=w252, y=w254) -> (x >= y?=w264:bool)
                    n200 = In Range and Coerce(upper limit=w255, x=w253, lower limit=w254) -> (In Range?=w256:bool)  [unwired: 1 out]
                    n201 = In Range and Coerce(upper limit=w255, x=w252, lower limit=w254) -> (In Range?=w257:bool)  [unwired: 1 out]
                    n202 = Threshold 1D Array(2:w292, 3:w284) -> (0:w283:dbl)  [unwired: 1 in]
                    n203 = Split 1D Array(array=w284, index=w283) -> ()  [unwired: 2 out]
                    n204 = case shown="真" w256 {
                      frame False {
                        n205 = property on="位移区间最大压力(KN) 2" class="DigNum (严格)"("NumText.TextColor"=u32 16720402) -> ()  [unwired: 2 in, 2 out]
                      }
                      frame True {
                        n206 = property on="位移区间最大压力(KN) 2" class="DigNum (严格)"("NumText.TextColor"=u32 0) -> ()  [unwired: 2 in, 2 out]
                      }
                    }
                    n207 = case shown="假" w257 {
                      frame False {
                        n208 = property on="位移区间最小压力(KN) 2" class="DigNum (严格)"("NumText.TextColor"=u32 16720402) -> ()  [unwired: 2 in, 2 out]
                      }
                      frame True {
                        n209 = property on="位移区间最小压力(KN) 2" class="DigNum (严格)"("NumText.TextColor"=u32 0) -> ()  [unwired: 2 in, 2 out]
                      }
                    }
                    n210 = And(x=w259, y=w264) -> (x .and. y?=w265:bool)
                    n211 = Split 1D Array(array=w285, index=w283) -> (first subarray=w282:dbl[])  [unwired: 1 out]
                    n212 = And(x=w258, y=w265) -> (x .and. y?=w263:bool)
                    n213 = Array Max & Min(array=w282) -> (max value=→"位移区间最大压力(KN) 2":dbl, min value=→"位移区间最小压力(KN) 2":dbl)  [unwired: 2 out]
                    n214 = case shown="假" w263 {
                      tunnel: [cluster{u32, u32}[] [{16711680, 16711680}, {16711680, 16711680}, {16711680, 16711680}, {16711680, 16711680}] cluster{u32, u32}[] [{6618880, 6618880}, {6618880, 6618880}, {6618880, 6618880}, {6618880, 6618880}]] -> w262
                      frame False {
                        n215 = shared-variable "我的电脑\\180.lvlib\\备用3"(u16 2 ("备用1")) -> ()  [unwired: 1 in, 1 out]
                        n216 = local write "判定结果 3"(bool[][] [[TRUE, FALSE]] ("判定结果")) -> ()
                      }
                      frame True {
                        n217 = shared-variable "我的电脑\\180.lvlib\\备用3"(u16 1 ("备用1")) -> ()  [unwired: 1 in, 1 out]
                        n218 = local write "判定结果 3"(bool[][] [[TRUE, TRUE]] ("判定结果")) -> ()
                      }
                    }
                    n219 = property on="判定结果 2" class="Bool (严格)"("Colors [4]"=w262) -> ()  [unwired: 2 in, 2 out]
                  }
                  frame 100 {
                    n220 = stacked-sequence {
                      frame #0 {
                        w307 = cluster{u32, u32}[] [{12369084, 12369084}, {12369084, 12369084}, {12369084, 12369084}, {12369084, 12369084}]
                        w308 = u32 0
                        w309 = 0.0 ("压装最大位移(mm)")
                        n221 = global read "Global.vi" "Result"() -> (w305:refnum<vi>)
                        n222 = local write "压装最大位移(mm)"(w309) -> ()
                        n223 = local write "位移区间最小压力(KN)"(w309) -> ()
                        n224 = local write "位移区间最大压力(KN)"(w309) -> ()
                        n225 = local write "压装最大位移(mm) 2"(w309) -> ()
                        n226 = local write "位移区间最小压力(KN) 2"(w309) -> ()
                        n227 = local write "位移区间最大压力(KN) 2"(w309) -> ()
                        n228 = property on="位移区间最大压力(KN) 2" class="DigNum (严格)"("NumText.TextColor"=w308) -> ()  [unwired: 2 in, 2 out]
                        n229 = property on="位移区间最小压力(KN) 2" class="DigNum (严格)"("NumText.TextColor"=w308) -> ()  [unwired: 2 in, 2 out]
                        n230 = property on="压装最大位移(mm) 2" class="DigNum (严格)"("NumText.TextColor"=w308) -> ()  [unwired: 2 in, 2 out]
                        n231 = property on="位移区间最大压力(KN)" class="DigNum (严格)"("NumText.TextColor"=w308) -> ()  [unwired: 2 in, 2 out]
                        n232 = property on="位移区间最小压力(KN)" class="DigNum (严格)"("NumText.TextColor"=w308) -> ()  [unwired: 2 in, 2 out]
                        n233 = property on="压装最大位移(mm)" class="DigNum (严格)"("NumText.TextColor"=w308) -> ()  [unwired: 2 in, 2 out]
                        n234 = for {
                          N: 4 -> [_]
                          tunnel: [cluster{dbl[], dbl[]} {[], []}] -> w310 mode=indexing
                        }
                        n235 = property class="Tbl"(reference=w305, "Value"=string[][] []) -> ()  [unwired: 1 in, 2 out]
                        n236 = local write "力位移曲线 2"(w310) -> ()
                        n237 = local write "力位移曲线"(w310) -> ()
                        n238 = property on="判定结果" class="Bool (严格)"("Colors [4]"=w307) -> ()  [unwired: 2 in, 2 out]
                        n239 = property on="判定结果 2" class="Bool (严格)"("Colors [4]"=w307) -> ()  [unwired: 2 in, 2 out]
                      }
                      frame #1 {
                        n240 = local read "左工位判定框参数"() -> (w314:string[][])
                        n241 = Index Array(array=w314, index (row) #1=0 ("索引 (行)"), index (row) #2=1 ("索引 (行)"), index (row) #3=2 ("索引 (行)"), index (row) #4=3 ("索引 (行)")) -> (element #1=w331:string[], element #2=w326:string[], element #3=w325:string[], element #4=w324:string[])  [unwired: 4 in]
                        n242 = Index Array(array=w326, index=1 ("索引")) -> (element=w318:string)
                        n243 = Index Array(array=w331, index=1 ("索引")) -> (element=w319:string)
                        n244 = Index Array(array=w324, index=1 ("索引")) -> (element=w316:string)
                        n245 = Index Array(array=w325, index=1 ("索引")) -> (element=w317:string)
                        n246 = local read "力位移曲线"() -> (w315:cluster{dbl[], dbl[]}[])
                        n247 = Decimal String To Number(string=w318) -> (number=w322:i32)  [unwired: 2 in, 1 out]
                        n248 = Decimal String To Number(string=w319) -> (number=w323:i32)  [unwired: 2 in, 1 out]
                        n249 = Decimal String To Number(string=w316) -> (number=w321:i32)  [unwired: 2 in, 1 out]
                        n250 = Decimal String To Number(string=w317) -> (number=w320:i32)  [unwired: 2 in, 1 out]
                        n251 = for {
                          tunnel: [w342] -> w313 mode=indexing
                          tunnel: w315 -> [w341] mode=indexing
                          tunnel: w323 -> [w339]
                          tunnel: w322 -> [w338]
                          tunnel: w321 -> [w337]
                          tunnel: w320 -> [w336]
                          i -> [w340]
                          n252 = case shown="0" w340 {
                            tunnel: [w343 w348] -> w342
                            tunnel: w341 -> [w343 _]
                            tunnel: w339 -> [_ w347]
                            tunnel: w338 -> [_ w346]
                            tunnel: w337 -> [_ w345]
                            tunnel: w336 -> [_ w344]
                            frame Default {
                            }
                            frame 0 {
                              n253 = Build Array(w347, w347, w346, w346, w347) -> (w349:i32[])
                              n254 = Build Array(w344, w345, w345, w344, w344) -> (w350:i32[])
                              n255 = Bundle(w349, w350) -> (w348:cluster{i32[], i32[]})  [unwired: 1 in]
                            }
                          }
                        }
                        n256 = local write "力位移曲线"(w313) -> ()
                      }
                      frame #2 {
                        n257 = local read "右工位判定框参数"() -> (w351:string[][])
                        n258 = Index Array(array=w351, index (row) #1=0 ("索引 (行)"), index (row) #2=1 ("索引 (行)"), index (row) #3=2 ("索引 (行)"), index (row) #4=3 ("索引 (行)")) -> (element #1=w369:string[], element #2=w364:string[], element #3=w363:string[], element #4=w362:string[])  [unwired: 4 in]
                        n259 = Index Array(array=w364, index=1 ("索引")) -> (element=w356:string)
                        n260 = Index Array(array=w369, index=1 ("索引")) -> (element=w357:string)
                        n261 = Index Array(array=w362, index=1 ("索引")) -> (element=w354:string)
                        n262 = Index Array(array=w363, index=1 ("索引")) -> (element=w355:string)
                        n263 = local read "力位移曲线 2"() -> (w353:cluster{dbl[], dbl[]}[])
                        n264 = Decimal String To Number(string=w356) -> (number=w360:i32)  [unwired: 2 in, 1 out]
                        n265 = Decimal String To Number(string=w357) -> (number=w361:i32)  [unwired: 2 in, 1 out]
                        n266 = Decimal String To Number(string=w354) -> (number=w359:i32)  [unwired: 2 in, 1 out]
                        n267 = Decimal String To Number(string=w355) -> (number=w358:i32)  [unwired: 2 in, 1 out]
                        n268 = for {
                          tunnel: [w380] -> w352 mode=indexing
                          tunnel: w353 -> [w379] mode=indexing
                          tunnel: w361 -> [w377]
                          tunnel: w360 -> [w376]
                          tunnel: w359 -> [w375]
                          tunnel: w358 -> [w374]
                          i -> [w378]
                          n269 = case shown="0" w378 {
                            tunnel: [w381 w386] -> w380
                            tunnel: w379 -> [w381 _]
                            tunnel: w377 -> [_ w385]
                            tunnel: w376 -> [_ w384]
                            tunnel: w375 -> [_ w383]
                            tunnel: w374 -> [_ w382]
                            frame Default {
                            }
                            frame 0 {
                              n270 = Build Array(w385, w385, w384, w384, w385) -> (w387:i32[])
                              n271 = Build Array(w382, w383, w383, w382, w382) -> (w388:i32[])
                              n272 = Bundle(w387, w388) -> (w386:cluster{i32[], i32[]})  [unwired: 1 in]
                            }
                          }
                        }
                        n273 = local write "力位移曲线 2"(w352) -> ()
                      }
                    }
                  }
                  frame 200 {
                    n274 = stacked-sequence {
                      frame #0 {
                        n275 = Wait (ms)(milliseconds to wait=u32 500 ("等待时间（毫秒）")) -> ()  [unwired: 1 out]
                        n276 = call "浮动通知.vi"("通知内容"="报表生成中" ("Status")) -> ()  [unwired: 11 in]
                      }
                      frame #1 {
                      }
                    }
                    n277 = control-ref of="报表"() -> (w389:refnum<vi>)
                    n278 = shared-variable "我的电脑\\180.lvlib\\备用2"() -> (w392:u16)  [unwired: 1 in, 1 out]
                    n279 = shared-variable "我的电脑\\180.lvlib\\备用1"(u16 201 ("备用1")) -> ()  [unwired: 1 in, 1 out]
                    n280 = global write "Global.vi" "Result"(w389) -> ()
                    n281 = case shown="2" w392 {
                      tunnel: [_ w393 w424] -> w390
                      frame 0, Default {
                      }
                      frame 1 {
                        n282 = local read "位移区间最大压力(KN)"() -> (w405:dbl)
                        n283 = local read "位移区间最小压力(KN)"() -> (w400:dbl)
                        n284 = local read "压装最大位移(mm)"() -> (w404:dbl)
                        n285 = local read "左压装上限"() -> (w397:dbl)
                        n286 = local read "左压装下限"() -> (w396:dbl)
                        n287 = local read "左上限1"() -> (w402:dbl)
                        n288 = local read "左下限1"() -> (w401:dbl)
                        n289 = local read "左上限2"() -> (w399:dbl)
                        n290 = local read "左下限2"() -> (w398:dbl)
                        n291 = Number To Fractional String(number=w405) -> (F-format string=w414:string)  [unwired: 3 in]
                        n292 = Number To Fractional String(number=w402) -> (F-format string=w413:string)  [unwired: 3 in]
                        n293 = Number To Fractional String(number=w401) -> (F-format string=w408:string)  [unwired: 3 in]
                        n294 = Number To Fractional String(number=w400) -> (F-format string=w411:string)  [unwired: 3 in]
                        n295 = Number To Fractional String(number=w399) -> (F-format string=w410:string)  [unwired: 3 in]
                        n296 = Number To Fractional String(number=w398) -> (F-format string=w407:string)  [unwired: 3 in]
                        n297 = Number To Fractional String(number=w404) -> (F-format string=w403:string)  [unwired: 3 in]
                        n298 = Number To Fractional String(number=w397) -> (F-format string=w395:string)  [unwired: 3 in]
                        n299 = Number To Fractional String(number=w396) -> (F-format string=w394:string)  [unwired: 3 in]
                        n300 = Build Array(w414, w413, w408) -> (w412:string[])
                        n301 = Build Array(w411, w410, w407) -> (w409:string[])
                        n302 = Build Array(w403, w395, w394) -> (w406:string[])
                        n303 = Build Array(w412, w409, w406) -> (w393:string[][])
                      }
                      frame 2 {
                        n304 = local read "位移区间最大压力(KN) 2"() -> (w423:dbl)
                        n305 = local read "位移区间最小压力(KN) 2"() -> (w420:dbl)
                        n306 = local read "压装最大位移(mm) 2"() -> (w417:dbl)
                        n307 = local read "右位移上限"() -> (w416:dbl)
                        n308 = local read "右位移下限"() -> (w415:dbl)
                        n309 = local read "右上限1"() -> (w422:dbl)
                        n310 = local read "右下限1"() -> (w421:dbl)
                        n311 = local read "右上限2"() -> (w419:dbl)
                        n312 = local read "右下限2"() -> (w418:dbl)
                        n313 = Number To Fractional String(number=w423) -> (F-format string=w436:string)  [unwired: 3 in]
                        n314 = Number To Fractional String(number=w422) -> (F-format string=w435:string)  [unwired: 3 in]
                        n315 = Number To Fractional String(number=w421) -> (F-format string=w430:string)  [unwired: 3 in]
                        n316 = Number To Fractional String(number=w420) -> (F-format string=w433:string)  [unwired: 3 in]
                        n317 = Number To Fractional String(number=w419) -> (F-format string=w432:string)  [unwired: 3 in]
                        n318 = Number To Fractional String(number=w418) -> (F-format string=w429:string)  [unwired: 3 in]
                        n319 = Number To Fractional String(number=w417) -> (F-format string=w427:string)  [unwired: 3 in]
                        n320 = Number To Fractional String(number=w416) -> (F-format string=w426:string)  [unwired: 3 in]
                        n321 = Number To Fractional String(number=w415) -> (F-format string=w425:string)  [unwired: 3 in]
                        n322 = Build Array(w436, w435, w430) -> (w434:string[])
                        n323 = Build Array(w433, w432, w429) -> (w431:string[])
                        n324 = Build Array(w427, w426, w425) -> (w428:string[])
                        n325 = Build Array(w434, w431, w428) -> (w424:string[][])
                      }
                    }
                    n326 = local write "报表"(w390) -> ()
                  }
                  frame 201 {
                    n327 = stacked-sequence {
                      frame #0 {
                        n328 = shared-variable "我的电脑\\180.lvlib\\备用1"(u16 0 ("备用1")) -> ()  [unwired: 1 in, 1 out]
                        n329 = Wait (ms)(milliseconds to wait=u32 800 ("等待时间（毫秒）")) -> ()  [unwired: 1 out]
                        n330 = shared-variable "我的电脑\\Global.lvlib\\工位追溯码"() -> (w443:string)  [unwired: 1 in, 1 out]
                        n331 = call "Report_A131258.vi"("文件重命名"=TRUE, "文件名称"=w443, "布尔数组"="判定结果 3") -> ()  [unwired: 8 in, 1 out]
                      }
                      frame #1 {
                      }
                    }
                  }
                  frame 1000 {
                    n332 = stacked-sequence {
                      frame #0 {
                        n333 = shared-variable "我的电脑\\Global.lvlib\\传感器码"("" ("传感器码")) -> ()  [unwired: 1 in, 1 out]
                      }
                      frame #1 {
                        w447 = "请扫码！" ("通知内容")
                        n334 = global read "Global1.vi" "联机模式"() -> (w445:enum16{"单机", "追溯"})
                        n335 = call "浮动通知.vi"("通知内容"=w447) -> ()  [unwired: 11 in]
                        n336 = case shown="\"追溯\"" w445 {
                          frame "单机", Default {
                            n337 = shared-variable "我的电脑\\180.lvlib\\备用1"(u16 1001 ("备用1")) -> ()  [unwired: 1 in, 1 out]
                          }
                          frame "追溯" {
                            n338 = stacked-sequence {
                              frame #0 {
                                n339 = global read "Global1.vi" "联机模式"() -> (w468:enum16{"单机", "追溯"})
                                n340 = call "GetSQLstring.vi"("联机模式"=w468) -> ("错误输出"=w466:errorcluster, "连接字符串"=w467:string)  [unwired: 9 in]
                                n341 = Concatenate Strings("SELECT RESULT_VALUE FROM RESULT  WHERE DEVICE_ID = \n" ("table"), "'2'" ("字符串"), " AND CODE_ID=" ("字符串"), "'1'" ("字符串")) -> (w465:string)
                                n342 = call-poly <vilib>:"DB Tools Open Connection.vi"("error in (no error)"=w466, "connection information"=w467) -> ("error out"=w459:errorcluster, "connection reference"=w460:T5)  [unwired: 6 in]
                                n343 = call-poly <vilib>:"DB Tools Execute Query.vi"("error in (no error)"=w459, "SQL query"=w465, "connection reference"=w460) -> ("error out"=w463:errorcluster, "recordset reference"=w464:T6)  [unwired: 5 in]
                                n344 = call-poly <vilib>:"DB Tools Fetch Recordset Data.vi"("error in (no error)"=w463, "recordset reference"=w464) -> ("error out"=w454:errorcluster, "recordset data"=w462:variant[][])  [unwired: 3 in, 1 out]
                                n345 = Variant To Data(error in=w454, type=string[][] [], Variant=w462) -> (data=w453:string[][])  [unwired: 1 out]
                                n346 = Index Array(array=w453, index (row)=0 ("索引 (行)")) -> (element=w451:string[])  [unwired: 1 in]
                                n347 = Index Array(array=w451, index=0 ("索引 (行)")) -> (element=w449:string)
                                n348 = local write "CODE_ID"(w449) -> ()
                              }
                              frame #1 {
                                n349 = local read "CODE_ID"() -> (w469:string)
                                n350 = global read "Global1.vi" "联机模式"() -> (w488:enum16{"单机", "追溯"})
                                n351 = call "GetSQLstring.vi"("联机模式"=w488) -> ("错误输出"=w486:errorcluster, "连接字符串"=w487:string)  [unwired: 9 in]
                                n352 = Concatenate Strings("SELECT RESULT_VALUE FROM RESULT  WHERE DEVICE_ID = \n" ("table"), "'2'" ("字符串"), " AND CODE_ID=" ("字符串"), w469) -> (w485:string)
                                n353 = call-poly <vilib>:"DB Tools Open Connection.vi"("error in (no error)"=w486, "connection information"=w487) -> ("error out"=w479:errorcluster, "connection reference"=w480:T5)  [unwired: 6 in]
                                n354 = call-poly <vilib>:"DB Tools Execute Query.vi"("error in (no error)"=w479, "SQL query"=w485, "connection reference"=w480) -> ("error out"=w483:errorcluster, "recordset reference"=w484:T6)  [unwired: 5 in]
                                n355 = call-poly <vilib>:"DB Tools Fetch Recordset Data.vi"("error in (no error)"=w483, "recordset reference"=w484) -> ("error out"=w475:errorcluster, "recordset data"=w482:variant[][])  [unwired: 3 in, 1 out]
                                n356 = Variant To Data(error in=w475, type=string[][] [], Variant=w482) -> (data=w471:string[][])  [unwired: 1 out]
                                n357 = Index Array(array=w471, index (row)=0 ("索引 (行)")) -> (element=w473:string[])  [unwired: 1 in]
                                n358 = Index Array(array=w473, index=0 ("索引 (行)")) -> (element=w470:string)
                                n359 = case shown="\"OK\"" w470 {
                                frame "假", Default {
                                }
                                frame "OK" {
                                n360 = shared-variable "我的电脑\\180.lvlib\\备用1"(u16 1001 ("备用1")) -> ()  [unwired: 1 in, 1 out]
                                }
                                frame "NG" {
                                }
                                }
                              }
                            }
                          }
                        }
                        n361 = call "输入框.vi"("提示信息"=w447) -> ("条形码输出"=w446:string)
                        n362 = shared-variable "我的电脑\\Global.lvlib\\传感器码"(w446) -> ()  [unwired: 1 in, 1 out]
                      }
                    }
                  }
                  frame 1001 {
                    n363 = shared-variable "我的电脑\\Global.lvlib\\传感器码"() -> (w492:string)  [unwired: 1 in, 1 out]
                    n364 = String Length(string=w492) -> (length=w491:i32)
                    n365 = Greater?(x=w491, y=4) -> (0:w493:bool)
                    n366 = case shown="真" w493 {
                      frame False {
                      }
                      frame True {
                        n367 = shared-variable "我的电脑\\180.lvlib\\备用1"(u16 1002 ("备用1")) -> ()  [unwired: 1 in, 1 out]
                      }
                    }
                  }
                }
              }
            }
          }
          event "删除": Value Change {
            n368 = event-data() -> ("NewVal"=w495:bool)  [unwired: 1 in, 5 out]
            n369 = case shown="真" w495 {
              tunnel: w496 -> [_ w498]
              frame False {
              }
              frame True {
                n370 = Concatenate Strings("确认删除“", "请选择要删除的产品", "”吗？") -> (w500:string)
                n371 = Two Button Dialog(message=w500) -> (T button?=w499:bool)  [unwired: 2 in]
                n372 = case shown="真" w499 {
                  tunnel: w498 -> [_ w504]
                  tunnel: "请选择要删除的产品" -> [_ w503]
                  frame False {
                  }
                  frame True {
                    n373 = call <vilib>:"Open Config Data.vi"("configuration file path"=w504) -> ("error out"=w506:errorcluster, "refnum"=w509:T4)  [unwired: 8 in, 1 out]
                    n374 = call <vilib>:"Remove Section.vi"("section"=w503, "error in (no error)"=w506, "refnum"=w509) -> ("error out"=w508:errorcluster, "section exists?"=w505:bool, "refnum out"=w507:T4)  [unwired: 6 in]
                    n375 = call <vilib>:"Close Config Data.vi"("error in (no error)"=w508, "refnum"=w507) -> ()  [unwired: 8 in, 2 out]
                    n376 = case shown="真" w505 {
                      frame False {
                        n377 = One Button Dialog(message="删除失败！\n请确认产品存在！" ("消息")) -> ()  [unwired: 1 in, 1 out]
                      }
                      frame True {
                        n378 = One Button Dialog(message="删除成功！" ("消息")) -> ()  [unwired: 1 in, 1 out]
                      }
                    }
                  }
                }
              }
            }
          }
          event "确定": Value Change {
            n379 = event-data() -> ("NewVal"=w512:bool)  [unwired: 1 in, 5 out]
            n380 = case shown="真" w512 {
              frame False {
              }
              frame True {
                n381 = stacked-sequence {
                  seq-local: [w513 _ _ _ _ _] -> [_ _ _ _ _ _]
                  frame #0 {
                    n382 = local read "产品型号"() -> (w516:string)
                    n383 = shared-variable "我的电脑\\Global.lvlib\\产品型号"(w516) -> ()  [unwired: 1 in, 1 out]
                    n384 = String Subset(string=w516, offset (0)=u16 2 ("偏移量(0)"), length (rest)=u16 4 ("长度（剩余）")) -> (substring=w513:string)
                    n385 = Decimal String To Number(string=w513) -> ()  [unwired: 2 in, 2 out]
                  }
                  frame #1 {
                    n386 = local read "左工位坐标轴参数"() -> (w517:string[][])
                    n387 = Index Array(array=w517, index (row) #1=0 ("索引 (行)"), index (row) #2=1 ("索引 (行)"), index (row) #3=2 ("索引 (行)"), index (row) #4=3 ("索引 (行)")) -> (element #1=w533:string[], element #2=w528:string[], element #3=w527:string[], element #4=w526:string[])  [unwired: 4 in]
                    n388 = Index Array(array=w533, index=1 ("索引")) -> (element=w525:string)
                    n389 = Index Array(array=w528, index=1 ("索引")) -> (element=w523:string)
                    n390 = Index Array(array=w527, index=1 ("索引")) -> (element=w522:string)
                    n391 = Index Array(array=w526, index=1 ("索引")) -> (element=w521:string)
                    n392 = Decimal String To Number(string=w525) -> (number=w524:i32)  [unwired: 2 in, 1 out]
                    n393 = Decimal String To Number(string=w523) -> (number=w520:i32)  [unwired: 2 in, 1 out]
                    n394 = Decimal String To Number(string=w522) -> (number=w519:i32)  [unwired: 2 in, 1 out]
                    n395 = Decimal String To Number(string=w521) -> (number=w518:i32)  [unwired: 2 in, 1 out]
                    n396 = property on="力位移曲线" class="XYGraph (严格)"("XScale.Minimum"=w524) -> ()  [unwired: 2 in, 2 out]
                    n397 = property on="力位移曲线" class="XYGraph (严格)"("XScale.Maximum"=w520) -> ()  [unwired: 2 in, 2 out]
                    n398 = property on="力位移曲线" class="XYGraph (严格)"("YScale.Minimum"=w519) -> ()  [unwired: 2 in, 2 out]
                    n399 = property on="力位移曲线" class="XYGraph (严格)"("YScale.Maximum"=w518) -> ()  [unwired: 2 in, 2 out]
                  }
                  frame #2 {
                    n400 = local read "右工位坐标轴参数"() -> (w542:string[][])
                    n401 = Index Array(array=w542, index (row) #1=0 ("索引 (行)"), index (row) #2=1 ("索引 (行)"), index (row) #3=2 ("索引 (行)"), index (row) #4=3 ("索引 (行)")) -> (element #1=w554:string[], element #2=w549:string[], element #3=w548:string[], element #4=w547:string[])  [unwired: 4 in]
                    n402 = Index Array(array=w554, index=1 ("索引")) -> (element=w546:string)
                    n403 = Index Array(array=w549, index=1 ("索引")) -> (element=w545:string)
                    n404 = Index Array(array=w548, index=1 ("索引")) -> (element=w544:string)
                    n405 = Index Array(array=w547, index=1 ("索引")) -> (element=w543:string)
                    n406 = Decimal String To Number(string=w546) -> (number=w541:i32)  [unwired: 2 in, 1 out]
                    n407 = Decimal String To Number(string=w545) -> (number=w540:i32)  [unwired: 2 in, 1 out]
                    n408 = Decimal String To Number(string=w544) -> (number=w539:i32)  [unwired: 2 in, 1 out]
                    n409 = Decimal String To Number(string=w543) -> (number=w538:i32)  [unwired: 2 in, 1 out]
                    n410 = property on="力位移曲线 2" class="XYGraph (严格)"("XScale.Minimum"=w541) -> ()  [unwired: 2 in, 2 out]
                    n411 = property on="力位移曲线 2" class="XYGraph (严格)"("XScale.Maximum"=w540) -> ()  [unwired: 2 in, 2 out]
                    n412 = property on="力位移曲线 2" class="XYGraph (严格)"("YScale.Minimum"=w539) -> ()  [unwired: 2 in, 2 out]
                    n413 = property on="力位移曲线 2" class="XYGraph (严格)"("YScale.Maximum"=w538) -> ()  [unwired: 2 in, 2 out]
                  }
                  frame #3 {
                    n414 = local read "左工位判定框参数"() -> (w568:string[][])
                    n415 = Index Array(array=w568, index (row) #1=0 ("索引 (行)"), index (row) #2=1 ("索引 (行)"), index (row) #3=2 ("索引 (行)"), index (row) #4=3 ("索引 (行)")) -> (element #1=w576:string[], element #2=w571:string[], element #3=w570:string[], element #4=w569:string[])  [unwired: 4 in]
                    n416 = Index Array(array=w571, index=1 ("索引")) -> (element=w562:string)
                    n417 = Index Array(array=w576, index=1 ("索引")) -> (element=w563:string)
                    n418 = Index Array(array=w569, index=1 ("索引")) -> (element=w560:string)
                    n419 = Index Array(array=w570, index=1 ("索引")) -> (element=w561:string)
                    n420 = local read "力位移曲线"() -> (w581:cluster{dbl[], dbl[]}[])
                    n421 = Decimal String To Number(string=w562) -> (number=w566:i32)  [unwired: 2 in, 1 out]
                    n422 = Decimal String To Number(string=w563) -> (number=w567:i32)  [unwired: 2 in, 1 out]
                    n423 = Decimal String To Number(string=w560) -> (number=w565:i32)  [unwired: 2 in, 1 out]
                    n424 = Decimal String To Number(string=w561) -> (number=w564:i32)  [unwired: 2 in, 1 out]
                    n425 = for {
                      tunnel: [w588] -> w559 mode=indexing
                      tunnel: w581 -> [w587] mode=indexing
                      tunnel: w567 -> [w585]
                      tunnel: w566 -> [w584]
                      tunnel: w565 -> [w583]
                      tunnel: w564 -> [w582]
                      i -> [w586]
                      n426 = case shown="0" w586 {
                        tunnel: [w589 w594] -> w588
                        tunnel: w587 -> [w589 _]
                        tunnel: w585 -> [_ w593]
                        tunnel: w584 -> [_ w592]
                        tunnel: w583 -> [_ w591]
                        tunnel: w582 -> [_ w590]
                        frame Default {
                        }
                        frame 0 {
                          n427 = Build Array(w593, w593, w592, w592, w593) -> (w595:i32[])
                          n428 = Build Array(w590, w591, w591, w590, w590) -> (w596:i32[])
                          n429 = Bundle(w595, w596) -> (w594:cluster{i32[], i32[]})  [unwired: 1 in]
                        }
                      }
                    }
                    n430 = local write "力位移曲线"(w559) -> ()
                  }
                  frame #4 {
                    n431 = local read "右工位判定框参数"() -> (w597:string[][])
                    n432 = Index Array(array=w597, index (row) #1=0 ("索引 (行)"), index (row) #2=1 ("索引 (行)"), index (row) #3=2 ("索引 (行)"), index (row) #4=3 ("索引 (行)")) -> (element #1=w615:string[], element #2=w610:string[], element #3=w609:string[], element #4=w608:string[])  [unwired: 4 in]
                    n433 = Index Array(array=w610, index=1 ("索引")) -> (element=w602:string)
                    n434 = Index Array(array=w615, index=1 ("索引")) -> (element=w603:string)
                    n435 = Index Array(array=w608, index=1 ("索引")) -> (element=w600:string)
                    n436 = Index Array(array=w609, index=1 ("索引")) -> (element=w601:string)
                    n437 = local read "力位移曲线 2"() -> (w598:cluster{dbl[], dbl[]}[])
                    n438 = Decimal String To Number(string=w602) -> (number=w606:i32)  [unwired: 2 in, 1 out]
                    n439 = Decimal String To Number(string=w603) -> (number=w607:i32)  [unwired: 2 in, 1 out]
                    n440 = Decimal String To Number(string=w600) -> (number=w605:i32)  [unwired: 2 in, 1 out]
                    n441 = Decimal String To Number(string=w601) -> (number=w604:i32)  [unwired: 2 in, 1 out]
                    n442 = for {
                      tunnel: [w626] -> w599 mode=indexing
                      tunnel: w598 -> [w625] mode=indexing
                      tunnel: w607 -> [w623]
                      tunnel: w606 -> [w622]
                      tunnel: w605 -> [w621]
                      tunnel: w604 -> [w620]
                      i -> [w624]
                      n443 = case shown="0" w624 {
                        tunnel: [w627 w632] -> w626
                        tunnel: w625 -> [w627 _]
                        tunnel: w623 -> [_ w631]
                        tunnel: w622 -> [_ w630]
                        tunnel: w621 -> [_ w629]
                        tunnel: w620 -> [_ w628]
                        frame Default {
                        }
                        frame 0 {
                          n444 = Build Array(w631, w631, w630, w630, w631) -> (w633:i32[])
                          n445 = Build Array(w628, w629, w629, w628, w628) -> (w634:i32[])
                          n446 = Bundle(w633, w634) -> (w632:cluster{i32[], i32[]})  [unwired: 1 in]
                        }
                      }
                    }
                    n447 = local write "力位移曲线 2"(w599) -> ()
                  }
                  frame #5 {
                    w635 = "参数装载成功！" ("消息")
                    n448 = call "浮动通知.vi"("通知内容"=w635) -> ()  [unwired: 11 in]
                    n449 = One Button Dialog(message=w635) -> ()  [unwired: 1 in, 1 out]
                  }
                }
              }
            }
          }
          event "添加": Value Change {
            n450 = event-data() -> ("NewVal"=w638:bool)  [unwired: 1 in, 5 out]
            n451 = local read "请输入添加的产品名称"() -> (w639:string)
            n452 = call <vilib>:"Trim Whitespace.vi"("string"=w639) -> ("trimmed string"=w640:string)  [unwired: 1 in]
            n453 = White Space?(1:w640) -> (0:w641:bool)
            n454 = case shown="假" w641 {
              tunnel: w636 -> [w644 _]
              tunnel: w638 -> [w643 _]
              tunnel: w637 -> [w642 _]
              frame False {
                n455 = case shown="真" w643 {
                  tunnel: w644 -> [_ w646]
                  tunnel: w642 -> [_ w645]
                  frame False {
                  }
                  frame True {
                    n456 = for {
                      tunnel: w646 -> [w649] mode=indexing
                      tunnel: w645 -> [w648]
                      n457 = call "Read_Write ParaINI File.vi"("Mode"=enum16{"Read", "Write"}."Write", "Section"="请输入添加的产品名称", "Filepath"=w648, "Ctl Refnum"=w649) -> ()  [unwired: 7 in, 1 out]
                    }
                  }
                }
              }
              frame True {
                w651 = 64 items=["None"=0, "Hand, Error, Stop"=16, "Question"=32, "Exclamation, Warning"=48, "Asterisk, Information"=64] ("icon")
                w652 = 0 items=["OK", "OKCancel", "AbortRetryIgnore", "YesNoCancel", "YesNo", "RetryCancel"] ("buttons")
                n458 = call "信息框（标题、文本、图标）.vi"("icon"=w651, "buttons"=w652, "caption"="添加失败", "text"="请输入产品名称!") -> ()  [unwired: 6 in, 2 out]
              }
            }
          }
          event "产品型号": Value Change {
            n459 = event-data() -> ()  [unwired: 1 in, 6 out]
            n460 = stacked-sequence {
              tunnel: w655 -> [_ w658]
              tunnel: w656 -> [_ w657]
              frame #0 {
              }
              frame #1 {
                n461 = for {
                  tunnel: w658 -> [w661] mode=indexing
                  tunnel: w657 -> [w660]
                  n462 = local read "产品型号"() -> (w659:string)
                  n463 = call "Read_Write ParaINI File.vi"("Mode"=enum16{"Read", "Write"}."Read", "Section"=w659, "Filepath"=w660, "Ctl Refnum"=w661) -> ()  [unwired: 7 in, 1 out]
                }
              }
            }
          }
          event "退出": Value Change {
            n464 = event-data() -> ()  [unwired: 1 in, 6 out]
            n465 = control-ref of="本VI"() -> (w665:refnum<vi>)
            n466 = invoke class="VI" method="FP.Close"(reference=w665) -> (reference out=w663:refnum<vi>, error out=w664:errorcluster)  [unwired: 2 in, 1 out]
            n467 = Close Reference(reference=w663, error in (no error)=w664) -> ()  [unwired: 1 out]
          }
          event "更新": Value Change {
            n468 = event-data() -> ("NewVal"=w668:bool)  [unwired: 1 in, 5 out]
            n469 = case shown="真" w668 {
              tunnel: w667 -> [_ w671]
              tunnel: w666 -> [_ w670]
              frame False {
              }
              frame True {
                n470 = for {
                  tunnel: w671 -> [w676]
                  tunnel: w670 -> [w675] mode=indexing
                  tunnel: [w674] -> w669
                  n471 = local read "产品型号"() -> (w678:string)
                  n472 = call "Read_Write ParaINI File.vi"("Mode"=enum16{"Read", "Write"}."Write", "Section"=w678, "Filepath"=w676, "Ctl Refnum"=w675) -> ("error out"=w674:errorcluster)  [unwired: 7 in]
                }
                n473 = case shown="无错误" w669 {
                  frame No Error {
                    n474 = call "浮动通知.vi"("通知内容"="更新成功！") -> ()  [unwired: 11 in]
                  }
                  frame Error {
                    n475 = call "浮动通知.vi"("通知内容"="更新失败！") -> ()  [unwired: 11 in]
                  }
                }
              }
            }
          }
          event "请输入添加的产品名称": Value Change {
            n476 = event-data() -> ("NewVal"=w679:string)  [unwired: 1 in, 5 out]
            n477 = control-ref of="产品型号"() -> (w680:refnum<vi>)
            n478 = property on="属性节点" class="CmbBox"(reference=w680) -> ("Strings[]"=w681:string[])  [unwired: 1 in, 2 out]
            n479 = for {
              tunnel: w679 -> [w682]
              tunnel: w681 -> [w683] mode=indexing
              n480 = Equal?(x=w682, y=w683) -> (x = y?=w684:bool)
              n481 = case shown="真" w684 {
                tunnel: w682 -> [_ w685]
                frame False {
                }
                frame True {
                  n482 = stacked-sequence {
                    tunnel: w685 -> [w691 _]
                    frame #0 {
                      w686 = 64 items=["None"=0, "Hand, Error, Stop"=16, "Question"=32, "Exclamation, Warning"=48, "Asterisk, Information"=64] ("icon")
                      w687 = 0 items=["OK", "OKCancel", "AbortRetryIgnore", "YesNoCancel", "YesNo", "RetryCancel"] ("buttons")
                      n483 = Concatenate Strings("已经存在产品”" ("text"), w691, "“\n请勿重复添加！" ("字符串")) -> (w689:string)
                      n484 = call "信息框（标题、文本、图标）.vi"("icon"=w686, "buttons"=w687, "caption"="产品重复", "text"=w689) -> ()  [unwired: 6 in, 2 out]
                    }
                    frame #1 {
                      n485 = local write "请输入添加的产品名称"("" ("请输入添加的产品名称")) -> ()
                    }
                  }
                }
              }
            }
          }
          event Panel Close {
            n486 = event-data() -> ()  [unwired: 1 in, 4 out]
            n487 = global write "Global.vi" "程序关闭"(TRUE ("程序关闭")) -> ()
          }
          event "确定按钮": Value Change {
            n488 = event-data() -> ()  [unwired: 1 in, 6 out]
            n489 = vi-ref "User_manager.vi"() -> (w696:refnum<vi>)
            n490 = call "CallVI.vi"("VI引用"=w696, "状态"=T1."Maximized") -> ()  [unwired: 11 in, 3 out]
          }
        }
        n491 = global read "Global.vi" "程序关闭"() -> (w113:bool)
      }
    }
    frame #3 {
      n492 = global write "Global.vi" "程序关闭"(TRUE ("程序关闭")) -> ()
    }
  }
